vi "GINKGO - MTMP.vi"() -> ()   [LabVIEW 2015]
uses:
  Global Variable/GV_Z axis.vi
  Global Variable/GV_Lock State.vi
  <vilib>/FPGAPlugInAG/PXI-7854R/niLvFpga_Open_PXI-7854R.vi
  <vilib>/rvi/interface/common/dynamic/niFpgaDynamicAddResources.vi
  <vilib>/FPGAPlugInAG/PXIe-7962R/niLvFpga_Open_PXIe-7962R.vi
  <vilib>/FPGAPlugInAG/Dynamic/niLvFpga_Abort_Dynamic.vi
  <vilib>/FPGAPlugInAG/Dynamic/niLvFpga_Reset_Dynamic.vi
  <vilib>/rvi/interface/common/niFpgaWaitOnOcc.vi
  <vilib>/Utility/error.llb/Error Cluster From Error Code.vi
  <vilib>/FPGAPlugInAG/Dynamic/niLvFpga_Run_Dynamic.vi
  <vilib>/rvi/errors/niLvFpgaAdjustHostInterfaceError.vi
  <vilib>/FPGAPlugInAG/Dynamic/niLvFpga_Close_Dynamic.vi
  Controls/Save picture camera.vi
  <vilib>/rvi/interface/nirviOpenFPGA/nirviOpenFPGA.xnode
  FPGA Bitfiles/GINKGO-MTPM_7854R_FPGAControl5_ktnmj4hxrpw.lvbitx
  FPGA/FPGA Control.vi
  FPGA Bitfiles/GINKGO-MTPM_7962R_FPGA796xR3_DMzdrFahWxE.lvbitx
  FPGA/FPGA 796xR.vi
  <vilib>/rvi/interface/nirviMethod/nirviMethod.xnode
  <vilib>/rvi/interface/nirviReadWriteControl/nirviReadWriteControl.xnode
  <vilib>/rvi/interface/nirviCloseFPGA/nirviCloseFPGA.xnode
  <vilib>/rvi/interface/Simulation/niFpgaSimulationCallBeginRW.vi
  <vilib>/rvi/errors/niLvFpgaMergeErrorWithErrorCode.vi
  <vilib>/FPGAPlugInAG/Dynamic/niLvFpga_ReadFifo_Dynamic.vi
  <vilib>/FPGAPlugInAG/Dynamic/niLvFpga_StopFifo_Dynamic.vi
  <vilib>/vision/NI_Vision_Development_Module.lvlib
  <vilib>/FPGAPlugInAG/Dynamic/niLvFpga_WriteFifo_Dynamic.vi
  <vilib>/FPGAPlugInAG/Dynamic/niLvFpga_ConfigureFifo_Dynamic.vi
  NiFpgaLv.dll
  <vilib>/FPGAPlugInAG/Dynamic/niLvFpga_StartFifo_Dynamic.vi
  FPGA Bitfiles/GINKGO-MTPM_7853R_FPGAControl5_AQdVoJZ010M.lvbitx
  <vilib>/FPGAPlugInAG/PXI-7853R/niLvFpga_Open_PXI-7853R.vi
  FPGA Bitfiles/GINKGO-MTPM_7961R_FPGA796xR2_Co2ELON9TL0.lvbitx
  <vilib>/FPGAPlugInAG/PXIe-7961R/niLvFpga_Open_PXIe-7961R.vi
panel:
  out "波形图表":sgl(graph)=113.25391
  out "Power Stop":bool=TRUE
  in  "Rolling Queue Flag":bool=TRUE
  out "Total Data Out":u16=13612
  in  "Acq. Start":u16=38 caption="Phase" max=6000 step=1
  in  "Real Back Period":u16=5 min=1
  out "实际深度":u32=16777216
  in  "Map Max.":i32=10000 caption="Max."
  in  "Map Min.":i32=-1000 caption="Min."
  out "Scale Value":dbl=0.1 caption="X"
  out "Total Frames":u16=43366
  in  "Max. Min.":cluster{i32, i32}(slide)={2599, 200} scale=-1000.0..10000.0
  in  "16-bit Display Method":u32(ring)=14 caption="Display Method" items=["Full Dynamic"=12, "Given Range"=14]
  in  "Rolling Average":dbl=2.0 min=1.0 step=1.0
  in  "Rolling":bool=TRUE
  out "User Define Phase":u32=866
  out "Image":T1(plugin-control)
  in  "Controls":T2(tab)
  out "Offset value":i16=113
  in  "Read offset":bool
  in  "Start Device":bool
  in  "PMT Shutter Pow.":bool
  out "Overload Dis.":bool=TRUE
  in  "Pulse Number":enum16{"SP", "DP"}(ring)=enum."DP"
  in  "Mems Enable":bool
  out "中心偏移":i32
  in  "互相关点数":i32=5
  in  "Calculate Phase shift":bool
  in  "Wave":enum16{"Triangle", "Sine", "Ramp"}(ring)=enum."Sine"
  in  "Interval Dis.":sgl=0.00049965957 min=-10 max=50 format="%.4f"
  in  "stop z stage":bool
  in  "5V":bool
  in  "Voltage Level":dbl=15.0 format="%#.3p"
  in  "Voltage Level 2":dbl=-15.0 caption="Voltage Level" format="%#.3p"
  in  "Source:Output Enabled":bool
  out "Voltage Measurement 2":dbl=1.359809204859642e-05 caption="Voltage Measurement"
  out "Compliance/Limit Reached 2":bool caption="Compliance/Limit Reached"
  out "Voltage Measurement":i8
  out "Compliance/Limit Reached":bool
  in  "MEMS SLOW":dbl(slide)=240000.0 caption="Slow" min=0.0 max=1000000.0 step=100.0 scale=0.0..300000.0 scale format="%#_6p"
  in  "MEMS FAST":dbl(slide) caption="Fast" min=0.0 max=1000000.0 step=100.0 scale=0.0..300000.0 scale format="%#_6p"
  out "Stimulate Time Dis.":u32
  in  "Stimulate Value":dbl=5.0 min=-10.0 max=10.0 format="%#_3f"
  in  "Stimulate Time":u32=500
  out "Stimulate Interval Time":dbl=0.9846153846153847
  in  "Stimulate Interval":u32=10
  in  "Stimulate Enable":bool caption="V.S."
  out "Frame Befor Time":dbl=422889087.50769234
  out "Frame Number":u32=4294967295
  in  "Frames Befor Stimulate":u32
  out "Acq. Sample Rate":dbl=120000000.0 caption="Sanple Rate Divider" format="%#_6p"
  in  "Microscope":enum16{"Miniature", "Benchtop"}(ring)
  in  "Line":u32(ring)=512 caption="Y" items=["8"=8, "16"=16, "32"=32, "64"=64, "128"=128, "256"=256, "512"=512, "1024"=1024, "2048"=2048]
  in  "X Offset":dbl caption="X" format="%#_3f"
  in  "Y Offset":dbl caption="Y" min=-10.0 max=10.0 format="%#_3f"
  in  "X Frequency":dbl(slide)=2600.0 caption="Speed" min=50.0 max=10000.0 step=1.0 scale=0.0..5000.0
  in  "Laser Intensity":dbl(slide)=1.5168539325842696 max=10.0 scale=0.0..5.0
  in  "Phase Shift":u32(slide)=868 caption="Phase" max=15000 step=2 scale=0.0..15000.0
  in  "Point":bool
  in  "PMT1 Sensitivity":dbl(slide)=0.6500000000000001 min=0.0 max=0.95 step=0.05 scale=0.0..0.95 scale format="%#_3f"
  in  "PMT1 Enable":bool
  out "Pixel Dwell":dbl=0.2988 format="%#_3g"
  out "Actual Positon":sgl=11.119017
  out "Actual Laser Intensity":dbl(knob)=9.99969482421875 scale=-10.0..1.0
  in  "PMT2 Switch":bool
  in  "PMT2 Sensitivity":dbl(slide)=0.45 min=0.0 max=0.95 step=0.05 scale=0.0..0.95 scale format="%#_3f"
  in  "File Name":string
  in  "Scale":bool
  in  "XY Home":bool
  in  "XY UP":bool
  in  "XY DOWN":bool
  in  "XY LEFT":bool
  in  "XY RIGHT":bool
  in  "Stop":bool=TRUE
  in  "LIVE":bool
  in  "Save":bool
  in  "Z-Stack":bool
  in  "Pixel/Line":u16(ring)=512 caption="X" items=["8"=8, "16"=16, "32"=32, "64"=64, "128"=128, "256"=256, "512"=512, "1024"=1024, "2048"=2048]
  in  "Gain":enum16{"0dB", "6dB", "12dB"}(ring)
  in  "Coulple":enum16{"AC", "DC"}(ring)=enum."DC"
  in  "Path":path=path "C:/Users/TVS001/Desktop/DATA/20180327-FHIRM TPM-2/26-Aglight-3" caption="Images Folder"
  out "Save Frames Dis.":u16=100
  in  "Save Frames":u16=100
  in  "ZOOM":u16(ring)=1 items=["User Define", "1X", "1.5X", "2X", "2.5X", "3X", "3.5X", "4X", "4.5X", "5X", "6X"]
  in  "Scan Mode":enum16{"Normal", "Line Scan", "Random Access"}(ring)
  in  "Y Amplitude":dbl=0.6 caption="Y" min=-10.0 max=18.0 format="%0.2p"
  in  "X Amplitude":dbl=0.6 caption="X" min=-10.0 max=18.0 format="%.2p"
  in  "Add Phase":bool
  in  "Move":bool=TRUE
  out "Frame Rate":dbl=10.15625 format="%#_3g"
  out "Ready":u8(slide)=10 scale=0.0..10.0
  in  "Z":bool
  out "Position":sgl=-5.9652176 format="%#_6f"
  in  "Set Zero":bool caption="空白按钮"
  in  "Reset Zero":bool caption="空白按钮"
  in  "Home Z":bool
  in  "Abs. Go":bool
  in  "Abs Pos X":sgl min=-10 max=360 format="%.6f"
  in  "Z Up":bool
  in  "Z Down":bool
  in  "Jog":sgl=0.0005 caption="Z" min=0 max=50 step=0.0001 format="%.4f"
  in  "Frames/Slice":u16=5
  in  "Slices":u16=87
  out "End Dis.":sgl=0.043470383 format="%#_6f"
  out "Start Dis.":sgl format="%#_6f"
  in  "End":bool
  in  "Start":bool
  in  "Restart":bool
  in  "Interval Time":u32=150
  in  "Zoom Standard":dbl[][](array[numeric])=[[10.0, 10.0, 11251.0], [6.66, 6.66, 10603.0], [5.0, 5.0, 10394.0], [4.0, 4.0, 10394.0], [3.34, 3.34, 8602.0], [2.86, 2.86, 10394.0], [2.5, 2.5, 10394.0], [2.222, 2.222, 10394.0], [1.3, 1.3, 8294.0], [0.6, 0.6, 8296.0]]
  in  "Zoom Miniature":dbl[][](array[numeric])=[[14.0, 7.6, 868.0], [12.0, 7.0, 876.0], [9.0, 6.0, 876.0], [7.2, 5.6, 754.0], [5.0, 3.4, 738.0], [5.14, 4.0, 846.0], [4.0, 2.6, 858.0], [3.6, 2.0, 840.0], [3.2, 1.9, 872.0], [3.0, 1.9, 866.0]]
  out "Test Point 3":u32=227362
  out "Test Point":u32
  out "Point/Pixel":i32=36
  in  "Focus Flag":bool
  out "Queue Number":i32=2
  out "Initial Z":bool
  out "Initialization Done":bool=TRUE
  in  "Start Control":bool
  out "Memory":i32(slide) scale=0.0..5000.0
  in  "Resource Name":refnum<k15>="PXI1Slot6"
  in  "Channel Name":string="1" caption="Channel Name 1"
  in  "Current Limit":dbl=0.5 format="%.3p"
  in  "Voltage Level Range":dbl=20.0 format="%.5p"
  in  "Current Limit Range":dbl=1.0 format="%.3p"
  in  "Source Delay (Sec)":dbl=0.1 format="%.3p"
  in  "Channel Name 2":string="2"
  out "Current Measurement 2":dbl=-5.469513872563125e-06 caption="Current Measurement"
  out "Current Measurement":i16
  out "Actual DDS Ticks":u32=1
  out "Actual DDS Sample Freq":u32=279173
  in  "OUTPUT Value Ticks":u32=44
  in  "DDS Ticks":u32=1
  out "Actual OUTPUT Value Ticks":u32=44
  in  "Random 1D Array":fxp<+/-,32,16>[](array[numeric]) format="%.21g"
  in  "MG17Motor Z":refnum<k7>(container)
  out "Acq. Point Dis.":u16=32
  in  "Divide":enum16{"120M", "60M", "30M", "15M", "7.5M"}(ring)
  out "Nonlinear Acq.":bool=TRUE
  in  "Adapter Module User Data 1":u8
  in  "Adapter Module User Data 0":u8
  in  "Adapter Module User Command":u8=3
  in  "Apply":bool
  in  "HWSerialNum":i32=49871607
  in  "Set Large Scale":dbl=0.5 caption="X"
  in  "Set Small Scale":dbl=0.1 caption="X"
  in  "Set Zero Value":sgl format="%#_6f"
  in  "Fill Fraction":dbl=0.8 min=0.1 max=6.0 step=0.01
  in  "Back Period":u16=5 min=1
  in  "Initial Benchtop Speed":dbl=500.0 caption="Speed" min=50.0 max=10000.0 step=1.0
  in  "Initial Miniature Speed":dbl=2600.0 caption="Speed" min=50.0 max=10000.0 step=1.0
  out "Acq.Point Array":u16[](graph)=[38, 38, 38, 37, 37, 37, 37, 36, 36, 36, 36, 36, 35, 35, 35, 35, 35, 34, 34, 34, 34, 34, 34, 33, 33, 33, 33, 33, 33, 32, 32, 32, 32, 32, 32, 32, 32, 31, 31, 31, 31, 31, 31, 31, 31, 30, 30, 30, 30, 30, 30, 30, 30, 30, 30, 29, 29, 29, 29, 29, 29, 29, 29, 29, 29, 29, 28, 28, 28, 28, 28, 28, 28, 28, 28, 28, 28, 28, 28, 28, 27, 27, 27, 27, 27, 27, 27, 27, 27, 27, 27, 27, 27, 27, 27, 27, 26, 26, 26, 26, 26, 26, 26, 26, 26, 26, 26, 26, 26, 26, 26, 26, 26, 26, 26, 26, 26, 25, 25, 25, 25, 25, 25, 25, 25, 25, 25, 25, 25, 25, 25, 25, 25, 25, 25, 25, 25, 25, 25, 25, 25, 25, 25, 25, 24, 24, 24, 24, 24, 24, 24, 24, 24, 24, 24, 24, 24, 24, 24, 24, 24, 24, 24, 24, 24, 24, 24, 24, 24, 24, 24, 24, 24, 24, 24, 24, 24, 24, 24, 24, 24, 24, 24, 24, 24, 24, 24, 23, 23, 23, 23, 23, 23, 23, 23, 23, 23, 23, 23, 23, 23, 23, 23, 23, 23, 23, 23, 23, 23, 23, 23, 23, 23, 23, 23, 23, 23, 23, 23, 23, 23, 23, 23, 23, 23, 23, 23, 23, 23, 23, 23, 23, 23, 23, 23, 23, 23, 23, 23, 23, 23, 23, 23, 23, 23, 23, 23, 23, 23, 23, 23, 23, 23, 23, 23, 23, 23, 23, 23, 23, 23, 23, 23, 23, 23, 23, 23, 23, 23, 23, 23, 23, 23, 23, 23, 23, 23, 23, 23, 23, 23, 23, 23, 23, 23, 23, 23, 23, 23, 23, 23, 23, 23, 23, 23, 23, 23, 23, 23, 23, 23, 23, 23, 23, 23, 23, 23, 23, 23, 23, 23, 23, 23, 23, 23, 23, 23, 23, 23, 23, 23, 23, 23, 23, 23, 24, 24, 24, 24, 24, 24, 24, 24, 24, 24, 24, 24, 24, 24, 24, 24, 24, 24, 24, 24, 24, 24, 24, 24, 24, 24, 24, 24, 24, 24, 24, 24, 24, 24, 24, 24, 24, 24, 24, 24, 24, 24, 24, 25, 25, 25, 25, 25, 25, 25, 25, 25, 25, 25, 25, 25, 25, 25, 25, 25, 25, 25, 25, 25, 25, 25, 25, 25, 25, 25, 26, 26, 26, 26, 26, 26, 26, 26, 26, 26, 26, 26, 26, 26, 26, 26, 26, 26, 26, 26, 26, 27, 27, 27, 27, 27, 27, 27, 27, 27, 27, 27, 27, 27, 27, 27, 27, 28, 28, 28, 28, 28, 28, 28, 28, 28, 28, 28, 28, 28, 28, 29, 29, 29, 29, 29, 29, 29, 29, 29, 29, 29, 30, 30, 30, 30, 30, 30, 30, 30, 30, 30, 31, 31, 31, 31, 31, 31, 31, 31, 32, 32, 32, 32, 32, 32, 32, 32, 33, 33, 33, 33, 33, 33, 34, 34, 34, 34, 34, 34, 35, 35, 35, 35, 35, 36, 36, 36, 36, 36, 37, 37, 37, 37, 38, 38, 38]
  out "Init Data Out":u16[](array[numeric])=[38, 38, 38, 37, 37, 37, 37, 36, 36, 36, 36, 36, 35, 35, 35, 35, 35, 34, 34, 34, 34, 34, 34, 33, 33, 33, 33, 33, 33, 32, 32, 32, 32, 32, 32, 32, 32, 31, 31, 31, 31, 31, 31, 31, 31, 30, 30, 30, 30, 30, 30, 30, 30, 30, 30, 29, 29, 29, 29, 29, 29, 29, 29, 29, 29, 29, 28, 28, 28, 28, 28, 28, 28, 28, 28, 28, 28, 28, 28, 28, 27, 27, 27, 27, 27, 27, 27, 27, 27, 27, 27, 27, 27, 27, 27, 27, 26, 26, 26, 26, 26, 26, 26, 26, 26, 26, 26, 26, 26, 26, 26, 26, 26, 26, 26, 26, 26, 25, 25, 25, 25, 25, 25, 25, 25, 25, 25, 25, 25, 25, 25, 25, 25, 25, 25, 25, 25, 25, 25, 25, 25, 25, 25, 25, 24, 24, 24, 24, 24, 24, 24, 24, 24, 24, 24, 24, 24, 24, 24, 24, 24, 24, 24, 24, 24, 24, 24, 24, 24, 24, 24, 24, 24, 24, 24, 24, 24, 24, 24, 24, 24, 24, 24, 24, 24, 24, 24, 23, 23, 23, 23, 23, 23, 23, 23, 23, 23, 23, 23, 23, 23, 23, 23, 23, 23, 23, 23, 23, 23, 23, 23, 23, 23, 23, 23, 23, 23, 23, 23, 23, 23, 23, 23, 23, 23, 23, 23, 23, 23, 23, 23, 23, 23, 23, 23, 23, 23, 23, 23, 23, 23, 23, 23, 23, 23, 23, 23, 23, 23, 23, 23, 23, 23, 23, 23, 23, 23, 23, 23, 23, 23, 23, 23, 23, 23, 23, 23, 23, 23, 23, 23, 23, 23, 23, 23, 23, 23, 23, 23, 23, 23, 23, 23, 23, 23, 23, 23, 23, 23, 23, 23, 23, 23, 23, 23, 23, 23, 23, 23, 23, 23, 23, 23, 23, 23, 23, 23, 23, 23, 23, 23, 23, 23, 23, 23, 23, 23, 23, 23, 23, 23, 23, 23, 23, 23, 24, 24, 24, 24, 24, 24, 24, 24, 24, 24, 24, 24, 24, 24, 24, 24, 24, 24, 24, 24, 24, 24, 24, 24, 24, 24, 24, 24, 24, 24, 24, 24, 24, 24, 24, 24, 24, 24, 24, 24, 24, 24, 24, 25, 25, 25, 25, 25, 25, 25, 25, 25, 25, 25, 25, 25, 25, 25, 25, 25, 25, 25, 25, 25, 25, 25, 25, 25, 25, 25, 26, 26, 26, 26, 26, 26, 26, 26, 26, 26, 26, 26, 26, 26, 26, 26, 26, 26, 26, 26, 26, 27, 27, 27, 27, 27, 27, 27, 27, 27, 27, 27, 27, 27, 27, 27, 27, 28, 28, 28, 28, 28, 28, 28, 28, 28, 28, 28, 28, 28, 28, 29, 29, 29, 29, 29, 29, 29, 29, 29, 29, 29, 30, 30, 30, 30, 30, 30, 30, 30, 30, 30, 31, 31, 31, 31, 31, 31, 31, 31, 32, 32, 32, 32, 32, 32, 32, 32, 33, 33, 33, 33, 33, 33, 34, 34, 34, 34, 34, 34, 35, 35, 35, 35, 35, 36, 36, 36, 36, 36, 37, 37, 37, 37, 38, 38, 38]
  out "x amp. new":dbl
  out "y amp. new":dbl
  in  "Add Random Access":bool
  out "x offset new":i16=-7638
  out "y offset new":i16=-4030
  in  "All Random Array":fxp<+/-,32,16>[][](array[numeric])
  in  "Clear Array":bool
  out "Random Phase":u32=12 caption="Phase" max=6000 step=1
  # "File Name"
  # "File Path"
  # "Save Frames"
  # "Microscope"
  # "Scan Mode"
  # "PMT1"
  # "PMT2"
  # "Frame Size"
  # "Gain"
  # "Scan Speed"
  # "Hz"
  # "V"
  # "V"
  # "Rate"
  # "Frame Rate"
  # "μs"
  # "Hz"
  # "Pixel Dwell"
  # "XY"
  # "Z"
  # "Zoom"
  # "Point"
  # "Amplitude"
  # "V"
  # "V"
  # "Phase"
  # "Laser"
  # "Intensity Map"
  # "Recent Z"
  # "Frames Before"
  # "s"
  # "Stimulate Interval"
  # "s"
  # "ms"
  # "Stimulate Time"
  # "V"
  # "Stimulate Intensity"
  # "Mode Switch"
  # "MEMS Filter"
  # "Acquisition Mode"
  # "Image Settings"
  # "Magnification"
  # "Save Settings"
  # "Position Settings"
  # "Detection Settings"
  # "Z-scan Settings"
  # "Vision Stimulate Settings"
  # "X"
  # "Y"
  # "Phase"
  # "1X"
  # "1.5X"
  # "2X"
  # "2.5X"
  # "3X"
  # "3.5X"
  # "4X"
  # "4.5X"
  # "5X"
  # "6X"
  # "X"
  # "Y"
  # "Phase"
  # "1X"
  # "1.5X"
  # "2X"
  # "2.5X"
  # "3X"
  # "3.5X"
  # "4X"
  # "4.5X"
  # "5X"
  # "6X"
  # "40859011"
  # "83856379"
  # "AO0 -- X-Miniature  \nAO1 -- Y-Miniature\nAO2 -- Laser Intensity\nAO3 -- PMT1\nAO4 -- PMT2 \nAO5 -- \nAO6 -- X-Benchtop\nAO7 -- Y-Benchtop\n\nAI0  -- Actual Laser Intensity"
  # "DIO0 -- Acqusition  \nDIO1 -- VSYNC\nDIO2 -- HSYNC \nDIO3 -- Laser Shutter\nDIO4 -- MEMS FAST Filter\nDIO5 -- MEMS SLOW Filter\nDIO6 -- PMT Shutter\nDIO7 -- PMT Shutter Pow.\nDIO8 -- Shock Detection \nDIO9 -- Foot-plate LIVE Detection"
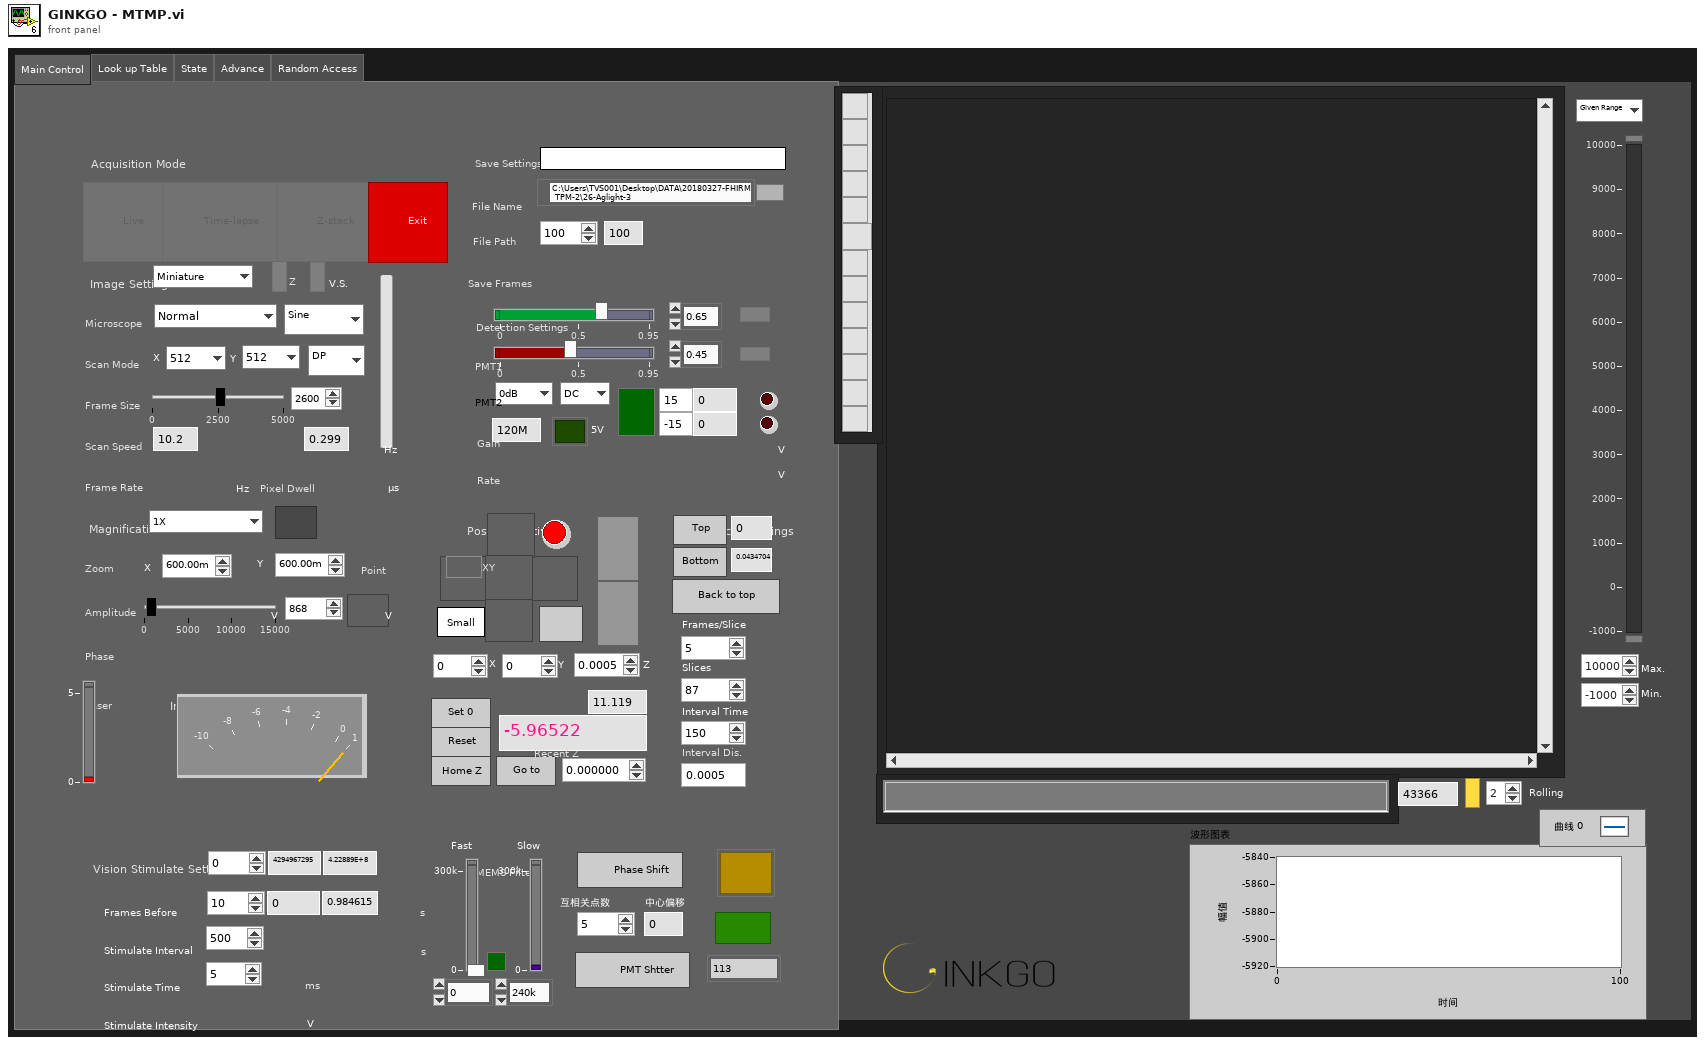
[diagram p1: front panel]
types:
  T1 = typedef "IMAQ Image.ctl" = refnum<image>
  T2 = enum32{"Main Control", "Look up Table", "State", "Advance", "Random Access"}
  T3 = typedef "Image Type" = u32
  T4 = enum8{"Enabled", "Disabled", "Disabled and Grayed Out"}
  T5 = cluster{"Global Rectangle":i32[], "Contours":cluster{"Contour Type":u32, "ROI Type":u32, "Points":i32[]}[]}
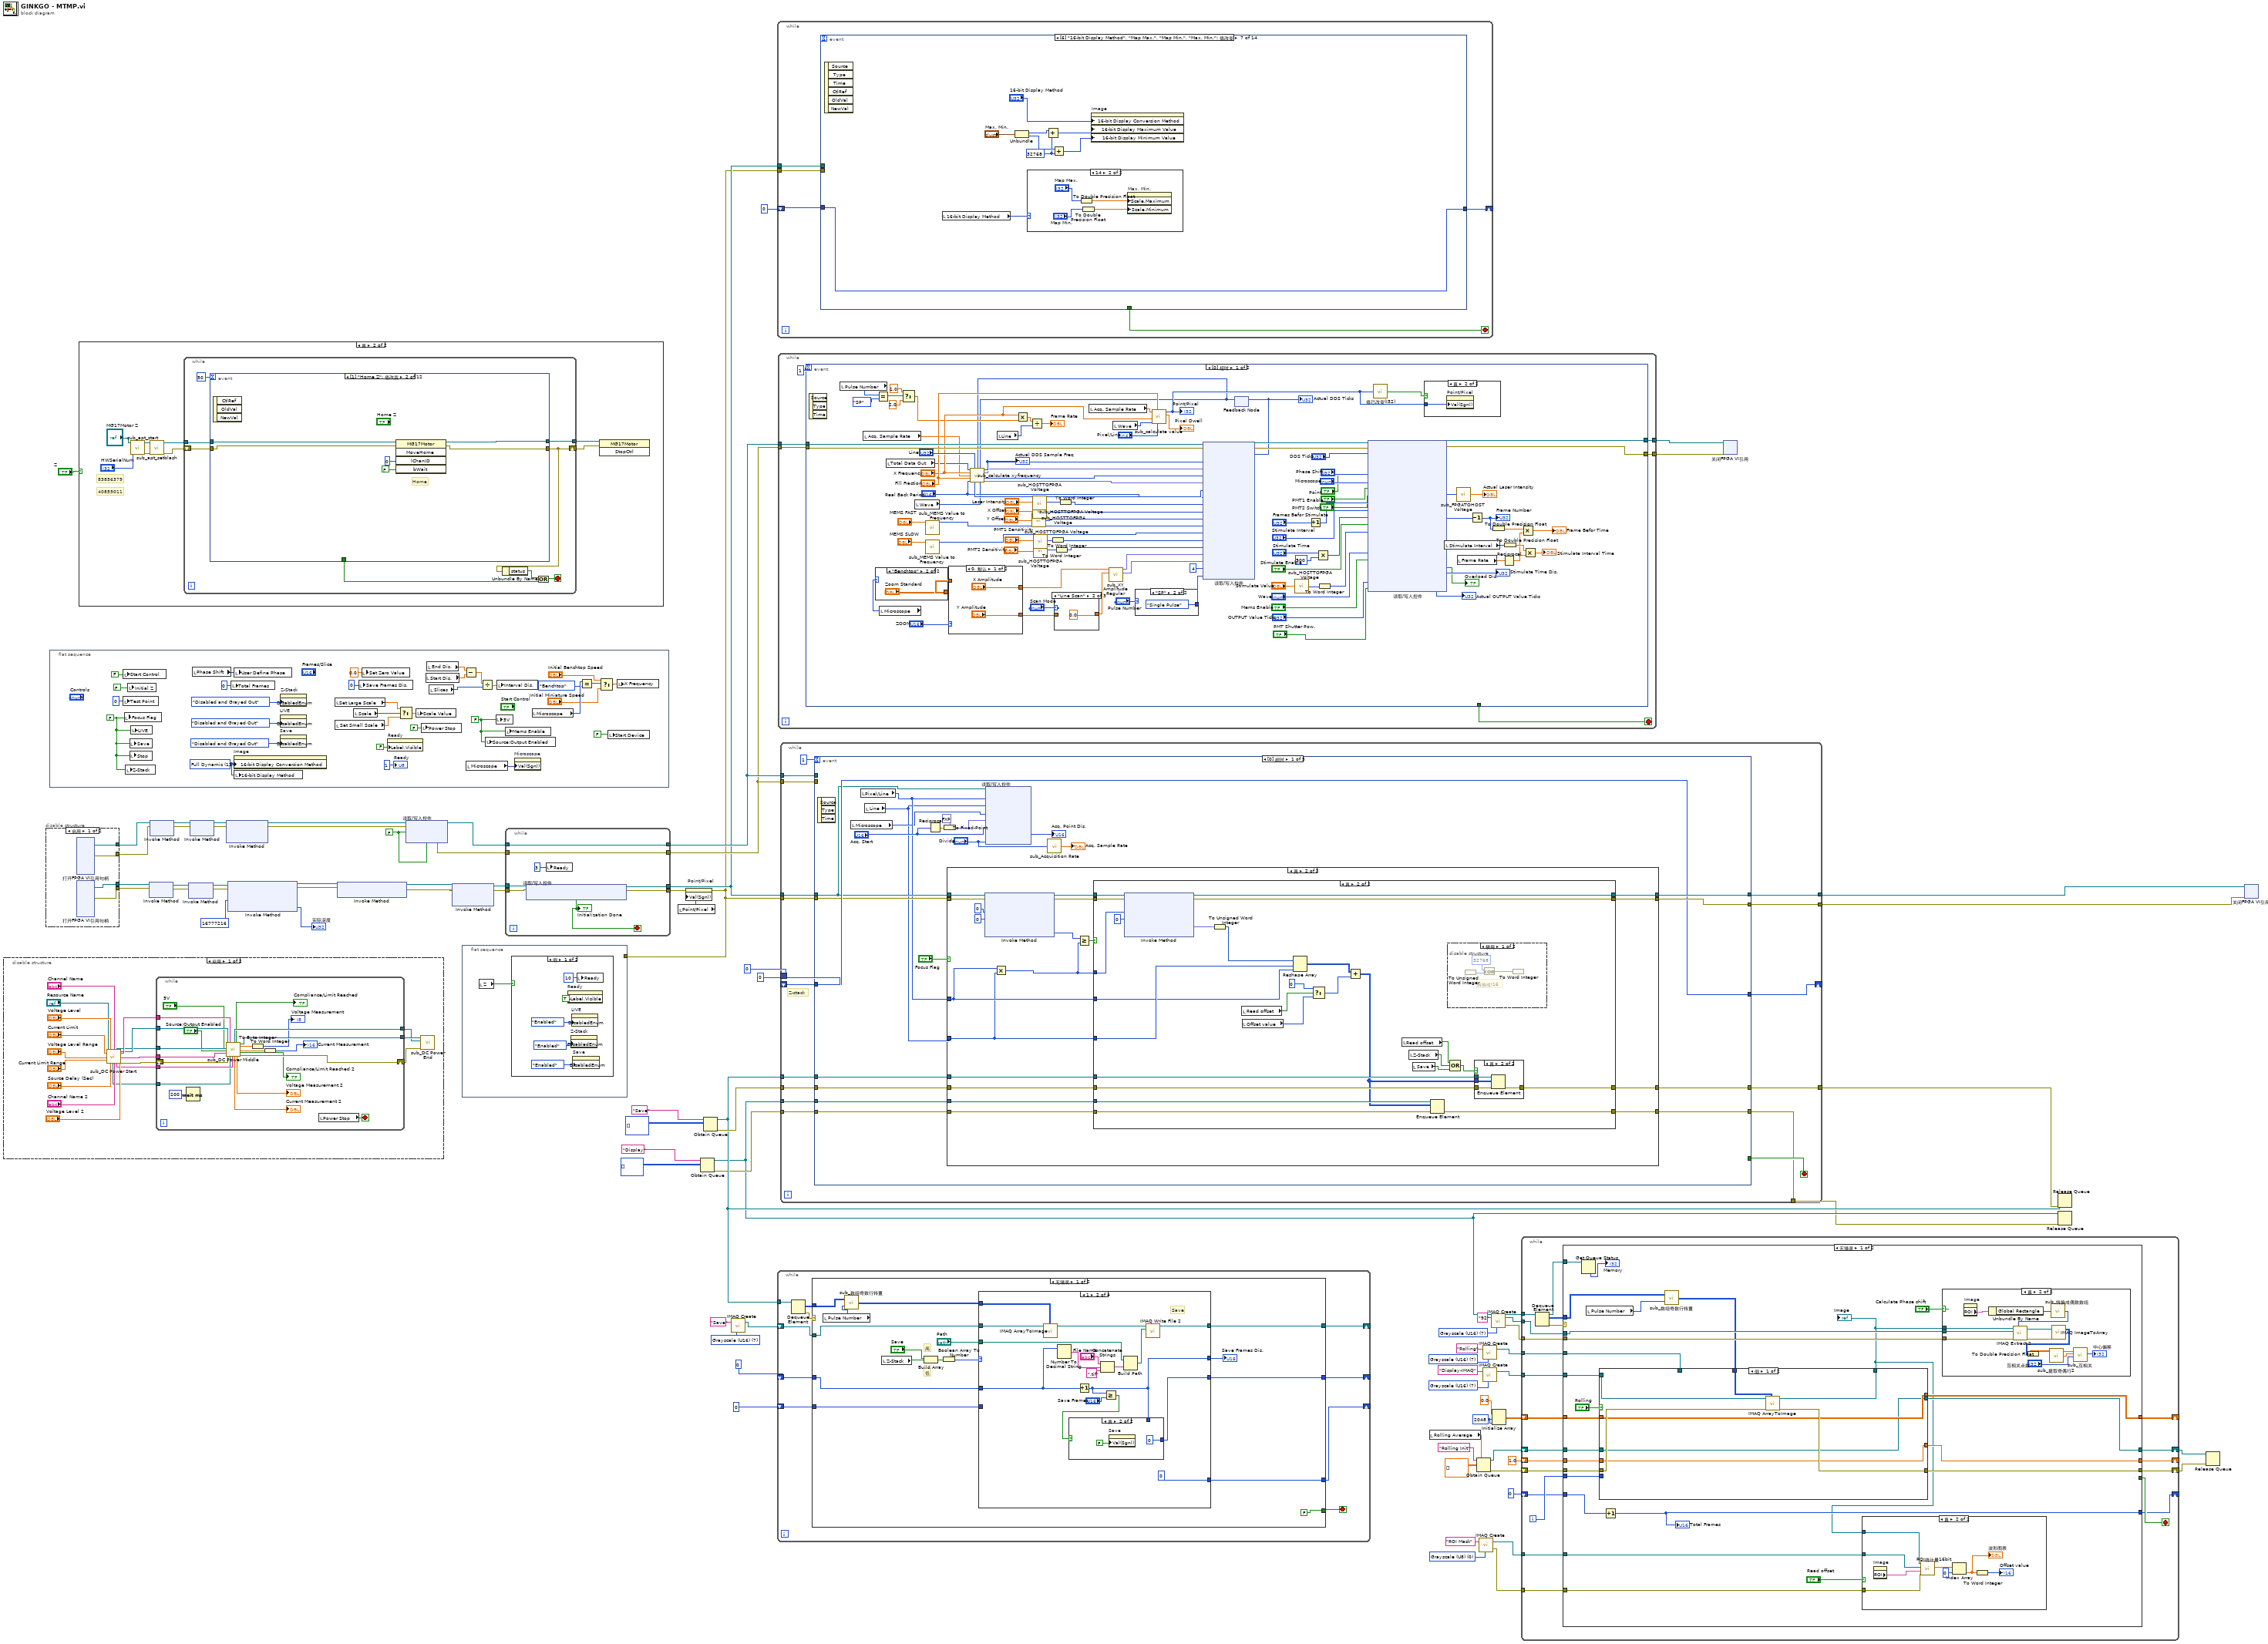
[diagram p0: block diagram]
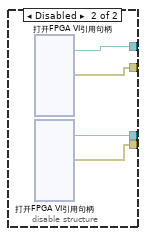
[diagram p2: hidden frame]
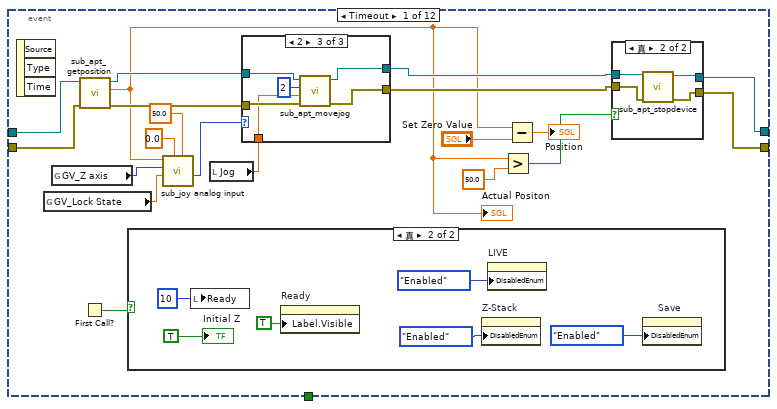
[diagram p4: hidden frame]
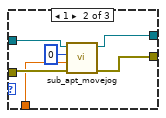
[diagram p6: hidden frame]
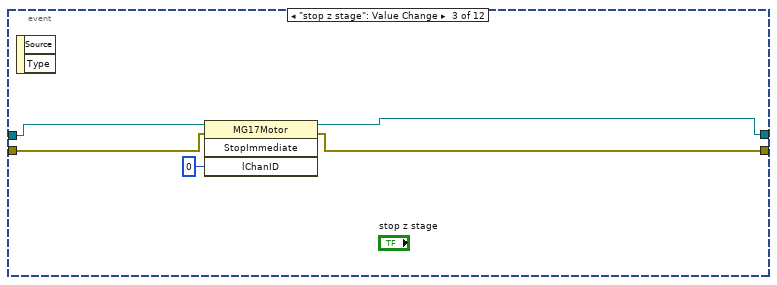
[diagram p9: hidden frame]
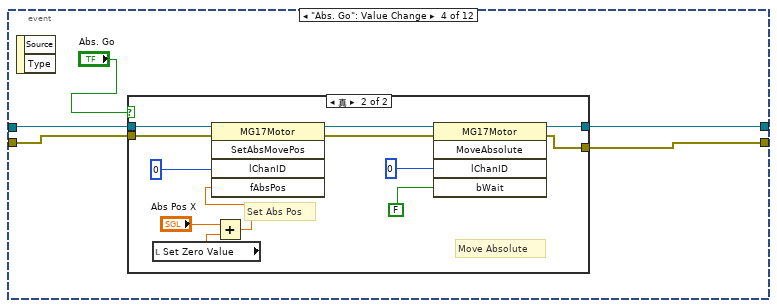
[diagram p10: hidden frame]
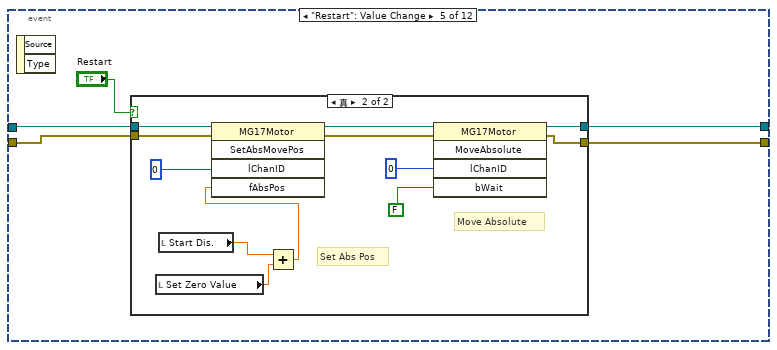
[diagram p12: hidden frame]
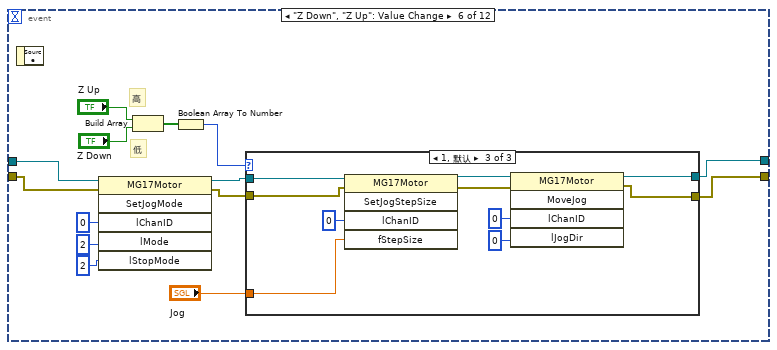
[diagram p14: hidden frame]
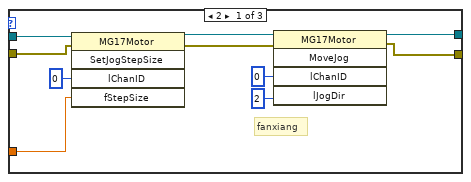
[diagram p15: hidden frame]
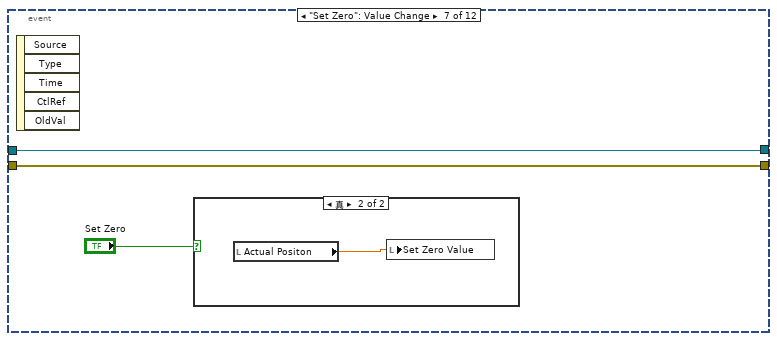
[diagram p17: hidden frame]
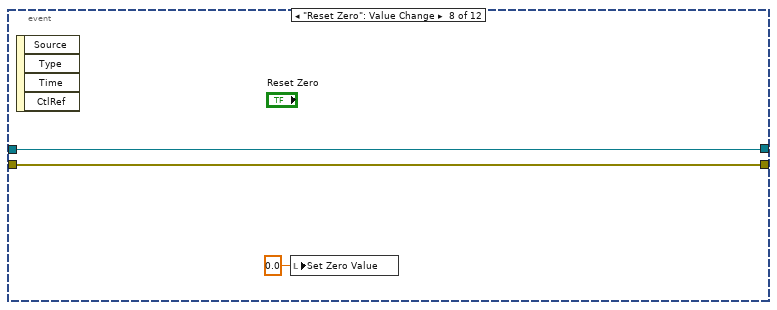
[diagram p19: hidden frame]
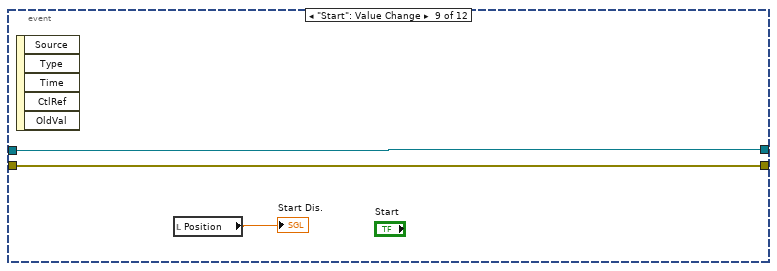
[diagram p20: hidden frame]
diagram:
  w3 = T3 0 items=["Grayscale (U8)", "Grayscale (I16)", "Grayscale (SGL)", "Complex (CSG)", "RGB (U32)", "HSL (U32)", "RGB (U64)", "Grayscale (U16)"] ("Image Type")
  w9 = T3 7 items=["Grayscale (U8)", "Grayscale (I16)", "Grayscale (SGL)", "Complex (CSG)", "RGB (U32)", "HSL (U32)", "RGB (U64)", "Grayscale (U16)"] ("Image Type")
  w15 = T3 7 items=["Grayscale (U8)", "Grayscale (I16)", "Grayscale (SGL)", "Complex (CSG)", "RGB (U32)", "HSL (U32)", "RGB (U64)", "Grayscale (U16)"] ("Image Type")
  w28 = T3 7 items=["Grayscale (U8)", "Grayscale (I16)", "Grayscale (SGL)", "Complex (CSG)", "RGB (U32)", "HSL (U32)", "RGB (U64)", "Grayscale (U16)"] ("Image Type")
  w38 = 2048 ("维数大小")
  w35 = T3 7 items=["Grayscale (U8)", "Grayscale (I16)", "Grayscale (SGL)", "Complex (CSG)", "RGB (U32)", "HSL (U32)", "RGB (U64)", "Grayscale (U16)"] ("Image Type")
  w49 = FALSE ("Enable")
  n1 = disable-structure shown="启用" {
    frame Enabled {
      n2 = call "sub_DC Power Start.vi"("IVI引用句柄输入"="Resource Name", "Current Limit"="Current Limit", "Voltage Level Range"="Voltage Level Range", "Current Limit Range"="Current Limit Range", "Voltage Level"="Voltage Level", "Source Delay (Sec)"="Source Delay (Sec)", "Channel Name"="Channel Name", "Channel Name 2"="Channel Name 2", "Voltage Level 2"="Voltage Level 2") -> ("instrument handle out 2"=w81:refnum<k15>, "instrument handle out"=w88:refnum<k15>, "Channel Name 6"=w82:string, "IVI引用句柄输出"=w96:refnum<k15>, "Channel Name 4"=w97:string, "Channel Name 3"=w90:string, "错误输出"=w87:errorcluster)  [unwired: 4 in]
      n3 = while {
        tunnel: w97 -> [w121]
        tunnel: w90 -> [w120]
        tunnel: [w119] -> w89
        shift-right: [w118] -> w86
        shift-left: w87 -> [w115]
        tunnel: w88 -> [w114]
        tunnel: w96 -> [w116]
        tunnel: [w117] -> w98
        tunnel: w82 -> [w104]
        tunnel: w81 -> [w103]
        stop <- w105 stop-if-true
        n4 = Wait (ms)(milliseconds to wait=u32 200 ("等待时间（毫秒）")) -> ()  [unwired: 1 out]
        n5 = call "sub_DC Power Middle.vi"("IVI引用句柄输入"=w116, "instrument handle out"=w114, "5V"="5V", "Source:Output Enabled"="Source:Output Enabled", "Channel Name 3"=w120, "错误输入（无错误）"=w115, "Channel Name 4"=w121, "instrument handle out 2"=w103, "Channel Name 5"=w104) -> ("instrument handle out 3"=w119:refnum<k15>, "Current Measurement 2"=→"Current Measurement 2":dbl, "Compliance/Limit Reached"=→"Compliance/Limit Reached":bool, "Voltage Measurement 2"=→"Voltage Measurement 2":dbl, "IVI引用句柄输出"=w117:refnum<k15>, "Voltage Measurement"=w111:dbl, "Current Measurement"=w110:dbl, "Compliance/Limit Reached 2"=→"Compliance/Limit Reached 2":bool, "错误输出"=w118:errorcluster)  [unwired: 2 in]
        n6 = To Byte Integer(number=w111) -> (8bit integer=→"Voltage Measurement":i8)
        n7 = To Word Integer(number=w110) -> (16bit integer=→"Current Measurement":i16)
        n8 = local read "Power Stop"() -> (w105:bool)
      }
      n9 = call "sub_DC Power End.vi"("错误输入（无错误）"=w86, "instrument handle out"=w89, "IVI引用句柄输入"=w98) -> ()  [unwired: 9 in]
    }
    frame Disabled {
    }
  }
  n10 = disable-structure shown="启用" {
    disable-tunnel: [w125 w129] -> w80
    disable-tunnel: [w124 w128] -> w79
    disable-tunnel: [w123 w126] -> w78
    disable-tunnel: [w122 w127] -> w77
    frame Enabled {
      n11 = xnode "打开FPGA VI引用句柄"() -> ("FPGA VI引用输出"=w125:refnum<k20>, "错误输出"=w124:errorcluster)  [unwired: 2 in]
      n12 = xnode "打开FPGA VI引用句柄"() -> ("FPGA VI引用输出"=w122:refnum<k20>, "错误输出"=w123:errorcluster)  [unwired: 2 in]
    }
    frame Disabled {
      n13 = xnode "打开FPGA VI引用句柄"() -> ("FPGA VI引用输出"=w129:refnum<k20>, "错误输出"=w128:errorcluster)  [unwired: 2 in]
      n14 = xnode "打开FPGA VI引用句柄"() -> ("FPGA VI引用输出"=w127:refnum<k20>, "错误输出"=w126:errorcluster)  [unwired: 2 in]
    }
  }
  n15 = flat-sequence {
    frame #0 {
      w144 = FALSE ("Focus")
      w152 = u32 12 items=["Default"=10, "Most Significant Bits"=11, "Full Dynamic"=12, "Downshift"=13, "Given Range"=14, "90% Dynamic"=15, "Given Percent Range"=16] ("16-bit Display Mapping:Conversion Method")
      w159 = FALSE ("Focus")
      n16 = local write "Start Control"(FALSE ("Initial")) -> ()
      n17 = local write "Test Point"(u32 0 ("Test Point")) -> ()
      n18 = local write "Focus Flag"(w159) -> ()
      n19 = local write "Z-Stack"(w159) -> ()
      n20 = local write "Initial Z"(FALSE ("Initial")) -> ()
      n21 = local write "Save"(w159) -> ()
      n22 = local write "Stop"(w159) -> ()
      n23 = local write "LIVE"(w159) -> ()
      n24 = local read "Phase Shift"() -> (w145:u32)
      n25 = local write "Total Frames"(u16 0 ("Total Frames")) -> ()
      n26 = property on="Image" class="ImageControl"("16-bit Display Conversion Method"=w152) -> ()  [unwired: 2 in, 2 out]
      n27 = local write "User Define Phase"(w145) -> ()
      n28 = local write "16-bit Display Method"(w152) -> ()
      n29 = property on="LIVE" class="Bool (严格)"("DisabledEnum"=T4."Disabled and Grayed Out" ("禁用")) -> ()  [unwired: 2 in, 2 out]
      n30 = property on="Save" class="Bool (严格)"("DisabledEnum"=T4."Disabled and Grayed Out" ("禁用")) -> ()  [unwired: 2 in, 2 out]
      n31 = property on="Z-Stack" class="Bool (严格)"("DisabledEnum"=T4."Disabled and Grayed Out" ("禁用")) -> ()  [unwired: 2 in, 2 out]
      n32 = local read "Set Large Scale"() -> (w151:dbl)
      n33 = local read "Set Small Scale"() -> (w150:dbl)
      n34 = local read "Scale"() -> (w149:bool)
      n35 = local write "Save Frames Dis."(u16 0 ("Save Frames Dis.")) -> ()
      n36 = local write "Set Zero Value"(sgl 0.0 ("Set Zero Value")) -> ()
      n37 = property on="Ready" class="Slide (严格)"("Label.Visible"=FALSE ("标签.可见")) -> ()  [unwired: 2 in, 2 out]
      n38 = Select(t=w151, s=w149, f=w150) -> (s? t:f=w148:dbl)
      n39 = local write "Scale Value"(w148) -> ()
      n40 = local write "Power Stop"(FALSE ("Power Stop")) -> ()
      n41 = local read "Start Dis."() -> (w141:sgl)
      n42 = local read "End Dis."() -> (w140:sgl)
      n43 = local read "Slices"() -> (w139:u16)
      n44 = Subtract(x=w140, y=w141) -> (x-y=w142:sgl)
      n45 = local read "Microscope"() -> (w138:enum16{"Miniature", "Benchtop"})
      n46 = Divide(x=w142, y=w139) -> (x/y=w143:sgl)
      n47 = local write "Source:Output Enabled"(w144) -> ()
      n48 = local write "5V"(w144) -> ()
      n49 = local write "Interval Dis."(w143) -> ()
      n50 = local write "Mems Enable"(w144) -> ()
      n51 = property on="Microscope" class="Enum (严格)"("Val(Sgnl)"=w138) -> ()  [unwired: 2 in, 2 out]
      n52 = local read "Microscope"() -> (w136:enum16{"Miniature", "Benchtop"})
      n53 = Equal?(x=w136, y=enum16{"Miniature", "Benchtop"}."Benchtop") -> (x = y?=w135:bool)
      n54 = Select(t="Initial Benchtop Speed", s=w135, f="Initial Miniature Speed") -> (s? t:f=w133:dbl)
      n55 = local write "Start Device"(FALSE ("Start Device")) -> ()
      n56 = local write "X Frequency"(w133) -> ()
      "Ready" <- u8 1 ("Process")
    }
  }
  n57 = case shown="真" "Z" {
    frame False {
    }
    frame True {
      # "40859011"
      # "83856379"
      n58 = call "sub_apt_start.vi"("HWSerialNum"="HWSerialNum", "引用"="MG17Motor Z") -> ("错误输出"=w167:errorcluster, "引用输出"=w168:refnum<k7>)  [unwired: 8 in]
      n59 = call "sub_apt_setblash.vi"("错误输入（无错误）"=w167, "引用"=w168) -> ("错误输出"=w165:errorcluster, "引用输出"=w166:refnum<k7>)  [unwired: 8 in]
      n60 = while {
        shift-right: [w174] -> w169
        shift-left: w165 -> [w177]
        tunnel: w166 -> [w178]
        tunnel: [w176] -> w170
        stop <- w172 stop-if-true
        n61 = event shown="[1] \"Home Z\": 值改变" {
          selector: _ -> [_ _ _ _ _ _ _ _ _ _ _ _]
          dyn-events: _ -> [_ _ _ _ _ _ _ _ _ _ _ _]
          timeout: 50 -> [_ _ _ _ _ _ _ _ _ _ _ _]
          tunnel: w178 -> [w191 w226 w234 w240 w259 w279 w312 w316 w319 w322 w325 w358]
          tunnel: w177 -> [w190 w225 w233 w239 w258 w278 w311 w315 w318 w321 w324 w357]
          tunnel: [w196 w228 w232 w238 w257 w287 w312 w316 w319 w322 w334 w358] -> w176
          tunnel: [w195 w227 w231 w237 w256 w286 w311 w315 w318 w321 w333 w357] -> w174
          tunnel: [_ _ _ _ _ _ _ _ _ _ _ TRUE ("Stop")] -> w171
          event Timeout {
            n62 = event-data() -> ()  [unwired: 1 in, 3 out]
            n63 = global read "GV_Lock State.vi" "GV_Lock State"() -> (w180:dbl)
            n64 = global read "GV_Z axis.vi" "GV_Z axis"() -> (w181:i32)
            n65 = call "sub_apt_getposition.vi"("错误输入（无错误）"=w190, "引用"=w191) -> ("错误输出"=w187:errorcluster, "GetPosition_Position"=w182:sgl, "引用输出"=w188:refnum<k7>)  [unwired: 7 in]
            "Actual Positon" <- w182
            n66 = First Call?() -> (First Call?: T/F=w194:bool)
            n67 = case shown="真" w194 {
              frame False {
              }
              frame True {
                n68 = local write "Ready"(u8 10 ("Process")) -> ()
                n69 = property on="Ready" class="Slide (严格)"("Label.Visible"=TRUE ("标签.可见")) -> ()  [unwired: 2 in, 2 out]
                n70 = property on="Z-Stack" class="Bool (严格)"("DisabledEnum"=T4."Enabled" ("禁用")) -> ()  [unwired: 2 in, 2 out]
                n71 = property on="LIVE" class="Bool (严格)"("DisabledEnum"=T4."Enabled" ("禁用")) -> ()  [unwired: 2 in, 2 out]
                n72 = property on="Save" class="Bool (严格)"("DisabledEnum"=T4."Enabled" ("禁用")) -> ()  [unwired: 2 in, 2 out]
                "Initial Z" <- TRUE ("Initial")
              }
            }
            n73 = call "sub_joy analog input.vi"("上限"=50.0 ("Displacement"), "下限"=0.0 ("Displacement"), "lock输入奇偶"=w180, "x"=w181, "Displacement"=w182) -> ("x state"=w183:i32)  [unwired: 5 in, 1 out]
            n74 = local read "Jog"() -> (w179:sgl)
            n75 = case shown="2" w183 {
              tunnel: [w200 w203 w209] -> w189
              tunnel: w188 -> [w200 w206 w212]
              tunnel: w187 -> [w199 w205 w211]
              tunnel: [w199 w204 w210] -> w186
              tunnel: w179 -> [_ w202 w208]
              frame 0, Default {
              }
              frame 1 {
                n76 = call "sub_apt_movejog.vi"("错误输入（无错误）"=w205, "Rel. Pos Y"=w202, "lJogDir"=0, "引用"=w206) -> ("error out"=w204:errorcluster, "MG17Motor Y"=w203:refnum<k7>)  [unwired: 6 in]
              }
              frame 2 {
                n77 = call "sub_apt_movejog.vi"("错误输入（无错误）"=w211, "Rel. Pos Y"=w208, "lJogDir"=2, "引用"=w212) -> ("error out"=w210:errorcluster, "MG17Motor Y"=w209:refnum<k7>)  [unwired: 6 in]
              }
            }
            n78 = Greater?(x=w182, y=sgl 50.0) -> (0:w197:bool)
            n79 = Subtract(x=w182, y="Set Zero Value") -> (x-y=→"Position":sgl)
            n80 = case shown="真" w197 {
              tunnel: w189 -> [w220 w224]
              tunnel: w186 -> [w219 w223]
              tunnel: [w220 w222] -> w196
              tunnel: [w219 w221] -> w195
              frame False {
              }
              frame True {
                n81 = call "sub_apt_stopdevice.vi"("错误输入（无错误）"=w223, "引用"=w224) -> ("错误输出"=w221:errorcluster, "引用输出"=w222:refnum<k7>)  [unwired: 8 in]
              }
            }
          }
          event "Home Z": Value Change {
            # "Home"
            n82 = event-data() -> ()  [unwired: 1 in, 3 out]
            n83 = invoke class="MG17Motor" method="MoveHome"(reference=w226, error in=w225, "lChanID"=0, "bWait"=FALSE) -> (reference out=w228:refnum<k7>, error out=w227:errorcluster)  [unwired: 1 in, 3 out]
          }
          event "stop z stage": Value Change {
            n84 = event-data() -> ()  [unwired: 1 in, 2 out]
            n85 = invoke class="MG17Motor" method="StopImmediate"(reference=w234, error in=w233, "lChanID"=0) -> (reference out=w232:refnum<k7>, error out=w231:errorcluster)  [unwired: 1 in, 2 out]
          }
          event "Abs. Go": Value Change {
            n86 = event-data() -> ()  [unwired: 1 in, 2 out]
            n87 = case shown="真" "Abs. Go" {
              tunnel: w240 -> [w242 w251]
              tunnel: w239 -> [w241 w250]
              tunnel: [w242 w247] -> w238
              tunnel: [w241 w246] -> w237
              frame False {
              }
              frame True {
                # "Set Abs Pos"
                # "Move Absolute"
                n88 = local read "Set Zero Value"() -> (w244:sgl)
                n89 = Add(x="Abs Pos X", y=w244) -> (x+y=w243:sgl)
                n90 = invoke class="MG17Motor" method="SetAbsMovePos"(reference=w251, error in=w250, "lChanID"=0, "fAbsPos"=w243) -> (reference out=w249:refnum<k7>, error out=w248:errorcluster)  [unwired: 1 in, 3 out]
                n91 = invoke class="MG17Motor" method="MoveAbsolute"(reference=w249, error in=w248, "lChanID"=0, "bWait"=FALSE) -> (reference out=w247:refnum<k7>, error out=w246:errorcluster)  [unwired: 1 in, 3 out]
              }
            }
          }
          event "Restart": Value Change {
            n92 = event-data() -> ()  [unwired: 1 in, 2 out]
            n93 = case shown="真" "Restart" {
              tunnel: w259 -> [w261 w270]
              tunnel: w258 -> [w260 w269]
              tunnel: [w261 w266] -> w257
              tunnel: [w260 w265] -> w256
              frame False {
              }
              frame True {
                # "Set Abs Pos"
                # "Move Absolute"
                n94 = local read "Set Zero Value"() -> (w264:sgl)
                n95 = local read "Start Dis."() -> (w263:sgl)
                n96 = Add(x=w263, y=w264) -> (x+y=w262:sgl)
                n97 = invoke class="MG17Motor" method="SetAbsMovePos"(reference=w270, error in=w269, "lChanID"=0, "fAbsPos"=w262) -> (reference out=w268:refnum<k7>, error out=w267:errorcluster)  [unwired: 1 in, 3 out]
                n98 = invoke class="MG17Motor" method="MoveAbsolute"(reference=w268, error in=w267, "lChanID"=0, "bWait"=FALSE) -> (reference out=w266:refnum<k7>, error out=w265:errorcluster)  [unwired: 1 in, 3 out]
              }
            }
          }
          event "Z Down", "Z Up": Value Change {
            # "低"
            # "高"
            n99 = event-data() -> ()  [unwired: 1 in, 1 out]
            n100 = invoke class="MG17Motor" method="SetJogMode"(reference=w279, error in=w278, "lChanID"=0, "lMode"=2, "lStopMode"=2) -> (reference out=w281:refnum<k7>, error out=w280:errorcluster)  [unwired: 1 in, 4 out]
            n101 = Build Array("Z Up", "Z Down") -> (w283:bool[])
            n102 = Boolean Array To Number(Boolean array=w283) -> (number=w282:u32)
            n103 = case shown="1, 默认" w282 {
              tunnel: w281 -> [w297 w299 w309]
              tunnel: [w295 w299 w307] -> w287
              tunnel: w280 -> [w292 w298 w304]
              tunnel: [w290 w298 w302] -> w286
              tunnel: "Jog" -> [w288 _ w300]
              frame 2 {
                # "fanxiang"
                n104 = invoke class="MG17Motor" method="SetJogStepSize"(reference=w297, error in=w292, "lChanID"=0, "fStepSize"=w288) -> (reference out=w296:refnum<k7>, error out=w291:errorcluster)  [unwired: 1 in, 3 out]
                n105 = invoke class="MG17Motor" method="MoveJog"(reference=w296, error in=w291, "lChanID"=0, "lJogDir"=2) -> (reference out=w295:refnum<k7>, error out=w290:errorcluster)  [unwired: 1 in, 3 out]
              }
              frame 0 {
              }
              frame 1, Default {
                n106 = invoke class="MG17Motor" method="SetJogStepSize"(reference=w309, error in=w304, "lChanID"=0, "fStepSize"=w300) -> (reference out=w308:refnum<k7>, error out=w303:errorcluster)  [unwired: 1 in, 3 out]
                n107 = invoke class="MG17Motor" method="MoveJog"(reference=w308, error in=w303, "lChanID"=0, "lJogDir"=0) -> (reference out=w307:refnum<k7>, error out=w302:errorcluster)  [unwired: 1 in, 3 out]
              }
            }
          }
          event "Set Zero": Value Change {
            n108 = event-data() -> ()  [unwired: 1 in, 5 out]
            n109 = case shown="真" "Set Zero" {
              frame False {
              }
              frame True {
                n110 = local read "Actual Positon"() -> (w313:sgl)
                n111 = local write "Set Zero Value"(w313) -> ()
              }
            }
          }
          event "Reset Zero": Value Change {
            n112 = event-data() -> ()  [unwired: 1 in, 4 out]
            n113 = local write "Set Zero Value"(sgl 0.0 ("Set Zero Value")) -> ()
          }
          event "Start": Value Change {
            n114 = event-data() -> ()  [unwired: 1 in, 5 out]
            n115 = local read "Position"() -> (→"Start Dis.":sgl)
          }
          event "End": Value Change {
            n116 = event-data() -> ()  [unwired: 1 in, 3 out]
            n117 = local read "Position"() -> (→"End Dis.":sgl)
          }
          event "Move": Value Change {
            n118 = event-data() -> ()  [unwired: 1 in, 1 out]
            n119 = invoke class="MG17Motor" method="SetJogMode"(reference=w325, error in=w324, "lChanID"=0, "lMode"=2, "lStopMode"=2) -> (reference out=w326:refnum<k7>, error out=w323:errorcluster)  [unwired: 1 in, 4 out]
            n120 = Absolute Value(x="Interval Dis.") -> (abs(x)=w330:sgl)
            n121 = Greater Than 0?(x="Interval Dis.") -> (x > 0?=w331:bool)
            n122 = case shown="假" w331 {
              tunnel: w326 -> [w346 w356]
              tunnel: [w344 w354] -> w334
              tunnel: w323 -> [w341 w351]
              tunnel: [w339 w349] -> w335
              tunnel: w330 -> [w337 w347]
              frame False {
                # "fanxiang"
                n123 = invoke class="MG17Motor" method="SetJogStepSize"(reference=w346, error in=w341, "lChanID"=0, "fStepSize"=w337) -> (reference out=w345:refnum<k7>, error out=w340:errorcluster)  [unwired: 1 in, 3 out]
                n124 = invoke class="MG17Motor" method="MoveJog"(reference=w345, error in=w340, "lChanID"=0, "lJogDir"=2) -> (reference out=w344:refnum<k7>, error out=w339:errorcluster)  [unwired: 1 in, 3 out]
              }
              frame True {
                n125 = invoke class="MG17Motor" method="SetJogStepSize"(reference=w356, error in=w351, "lChanID"=0, "fStepSize"=w347) -> (reference out=w355:refnum<k7>, error out=w350:errorcluster)  [unwired: 1 in, 3 out]
                n126 = invoke class="MG17Motor" method="MoveJog"(reference=w355, error in=w350, "lChanID"=0, "lJogDir"=0) -> (reference out=w354:refnum<k7>, error out=w349:errorcluster)  [unwired: 1 in, 3 out]
              }
            }
            n127 = property on="Z-Stack" class="Bool (严格)"(error in=w335, "Val(Sgnl)"=TRUE ("值(信号)")) -> (error out=w333:errorcluster)  [unwired: 1 in, 1 out]
          }
          event "Stop": Value Change {
            n128 = event-data() -> ()  [unwired: 1 in, 4 out]
          }
        }
        n129 = Unbundle By Name(w174) -> ("status"=w173:bool)
        n130 = Or(x=w173, y=w171) -> (x .or. y?=w172:bool)
      }
      n131 = invoke class="MG17Motor" method="StopCtrl"(reference=w170, error in=w169) -> ()  [unwired: 1 in, 3 out]
    }
  }
  n132 = xnode "Invoke Method"("FPGA VI引用输入"=w77, "错误输入"=w78) -> ("FPGA VI引用输出"=w66:refnum<k20>, "错误输出"=w67:errorcluster)
  n133 = xnode "Invoke Method"("FPGA VI引用输入"=w80, "错误输入"=w79) -> ("FPGA VI引用输出"=w63:refnum<k20>, "错误输出"=w62:errorcluster)
  n134 = xnode "Invoke Method"("FPGA VI引用输入"=w66, "错误输入"=w67) -> ("FPGA VI引用输出"=w68:refnum<k20>, "错误输出"=w69:errorcluster)
  n135 = xnode "Invoke Method"("FPGA VI引用输入"=w63, "错误输入"=w62) -> ("FPGA VI引用输出"=w61:refnum<k20>, "错误输出"=w60:errorcluster)
  n136 = xnode "Invoke Method"("FPGA VI引用输入"=w61, "错误输入"=w60) -> ("FPGA VI引用输出"=w59:refnum<k20>, "错误输出"=w58:errorcluster)  [unwired: 1 in]
  n137 = xnode "Invoke Method"("FPGA VI引用输入"=w68, "错误输入"=w69, "请求的深度"=u32 16777216) -> ("FPGA VI引用输出"=w65:refnum<k20>, "错误输出"=w64:errorcluster, "实际深度"=→"实际深度":u32)
  n138 = xnode "Invoke Method"("FPGA VI引用输入"=w65, "错误输入"=w64) -> ("FPGA VI引用输出"=w31:refnum<k20>, "错误输出"=w30:errorcluster)
  n139 = xnode "读取/写入控件"("FPGA VI引用输入"=w59, "错误输入"=w58, "Shutter"=w49, "Start Control"=w49) -> ("FPGA VI引用输出"=w51:refnum<k20>, "错误输出"=w50:errorcluster)
  n140 = xnode "Invoke Method"("FPGA VI引用输入"=w31, "错误输入"=w30) -> ("FPGA VI引用输出"=w55:refnum<k20>, "错误输出"=w54:errorcluster)  [unwired: 1 in]
  n141 = flat-sequence {
    tunnel: w5 -> [_]
    frame #0 {
      n142 = local read "Z"() -> (w360:bool)
      n143 = case shown="假" w360 {
        frame False {
          n144 = property on="Ready" class="Slide (严格)"("Label.Visible"=TRUE ("标签.可见")) -> ()  [unwired: 2 in, 2 out]
          n145 = property on="Z-Stack" class="Bool (严格)"("DisabledEnum"=T4."Enabled" ("禁用")) -> ()  [unwired: 2 in, 2 out]
          n146 = property on="LIVE" class="Bool (严格)"("DisabledEnum"=T4."Enabled" ("禁用")) -> ()  [unwired: 2 in, 2 out]
          n147 = property on="Save" class="Bool (严格)"("DisabledEnum"=T4."Enabled" ("禁用")) -> ()  [unwired: 2 in, 2 out]
          n148 = local write "Ready"(u8 10 ("Process")) -> ()
        }
        frame True {
          n149 = local write "Ready"(u8 6 ("Process")) -> ()
        }
      }
    }
  }
  n150 = while {
    tunnel: w55 -> [w374]
    tunnel: w54 -> [w373]
    tunnel: [w372] -> w19
    tunnel: [w371] -> w6
    tunnel: [w370] -> w52
    tunnel: w51 -> [w370]
    tunnel: [w369] -> w47
    tunnel: w50 -> [w369]
    stop <- w367 stop-if-true
    n151 = xnode "读取/写入控件"("FPGA VI引用输入"=w374, "错误输入"=w373) -> ("FPGA VI引用输出"=w372:refnum<k20>, "错误输出"=w371:errorcluster, "Adapter Module Initialization Done"=w367:bool)
    "Initialization Done" <- w367
    n152 = local write "Ready"(u8 3 ("Process")) -> ()
  }
  n153 = local read "Point/Pixel"() -> (w7:i32)
  n154 = property on="Point/Pixel" class="DigNum (严格)"(error in=w6, "Val(Sgnl)"=w7) -> (error out=w5:errorcluster)  [unwired: 1 in, 1 out]
  n155 = Obtain Queue(name (unnamed)="Display" ("名称（未命名）"), element data type=i16[][] []) -> (queue out=w21:refnum<queue>, error out=w22:errorcluster)  [unwired: 3 in, 1 out]
  n156 = Obtain Queue(name (unnamed)="Save" ("名称（未命名）"), element data type=i16[][] []) -> (queue out=w32:refnum<queue>, error out=w76:errorcluster)  [unwired: 3 in, 1 out]
  n157 = call "IMAQ Create"("Image Name"="Save", "Image Type"=w28) -> ("New Image"=w26:T1)  [unwired: 3 in, 1 out]
  n158 = while {
    tunnel: w32 -> [w384]
    shift-right: [w380] -> _
    shift-left: u16 0 -> [w381]
    shift-right: [w377] -> _
    shift-left: u16 0 -> [w378]
    shift-right: [w375] -> _
    shift-left: w26 -> [w379]
    stop <- w376 stop-if-true
    n159 = Dequeue Element(queue=w384) -> (element=w382:i16[][], error out=w383:errorcluster)  [unwired: 2 in, 2 out]
    n160 = case shown="无错误" w383 {
      tunnel: w382 -> [w388 _]
      tunnel: w381 -> [w400 w461]
      tunnel: [w399 w461] -> w380
      tunnel: w379 -> [w398 w458]
      tunnel: w378 -> [w391 w460]
      tunnel: [w390 w460] -> w377
      tunnel: [FALSE TRUE] -> w376
      tunnel: [w385 w458] -> w375
      frame No Error {
        # "高"
        # "低"
        n161 = local read "Pulse Number"() -> (w387:enum16{"SP", "DP"})
        n162 = call "sub_数组奇数行转置.vi"("Pulse Number"=w387, "Input"=w388) -> ("output"=w386:u16[][])
        n163 = local read "Z-Stack"() -> (w396:bool)
        n164 = Build Array("Save", w396) -> (w395:bool[])
        n165 = Boolean Array To Number(Boolean array=w395) -> (number=w394:u32)
        n166 = case shown="1" w394 {
          tunnel: w400 -> [w403 w420 w438 w456]
          tunnel: [u16 0 w419 w440 u16 0] -> w399
          tunnel: w398 -> [w401 w418 w443 w454]
          tunnel: w386 -> [_ w405 w424 _]
          tunnel: "Path" -> [_ w417 w442 _]
          tunnel: [w403 w416 w436 w456] -> w392
          tunnel: w391 -> [_ _ w437 _]
          tunnel: [u16 0 ("t") u16 0 ("t") w439 u16 0] -> w390
          tunnel: [w401 w406 w425 w454] -> w385
          frame 0, Default {
          }
          frame 1 {
            # "Save"
            n167 = call "IMAQ ArrayToImage"("Image Pixels (U16)"=w405, "Image"=w418) -> ("Image Out"=w408:T1)  [unwired: 8 in, 1 out]
            n168 = Number To Decimal String(number=w420) -> (decimal integer string=w413:string)  [unwired: 1 in]
            n169 = Increment(x=w420) -> (x+1=w416:u16)
            n170 = Concatenate Strings("File Name", w413, ".tif" ("字符串")) -> (w414:string)
            n171 = Greater Or Equal?(x=w416, y="Save Frames") -> (x >= y?=w409:bool)
            n172 = case shown="真" w409 {
              tunnel: [w421 u16 0] -> w419
              tunnel: w416 -> [w421 _]
              frame False {
              }
              frame True {
                n173 = property on="Save" class="Bool (严格)"("Val(Sgnl)"=FALSE ("Save")) -> ()  [unwired: 2 in, 2 out]
              }
            }
            n174 = Build Path(base path=w417, name or relative path=w414) -> (appended path=w411:path)
            n175 = call-poly "IMAQ Write File 2"("File Path"=w411, "Image"=w408) -> ("Image Out (duplicate)"=w406:T1)  [unwired: 8 in, 1 out]
          }
          frame 2 {
            # "Z-Stack"
            n176 = local read "Frames/Slice"() -> (w428:u16)
            n177 = call "IMAQ ArrayToImage"("Image Pixels (U16)"=w424, "Image"=w443) -> ("Image Out"=w430:T1)  [unwired: 8 in, 1 out]
            n178 = Multiply(x=w437, y=w428) -> (x*y=w429:u16)
            n179 = Add(x=w429, y=w438) -> (x+y=w427:u16)
            n180 = Increment(x=w438) -> (x+1=w441:u16)
            n181 = Number To Decimal String(number=w427) -> (decimal integer string=w433:string)  [unwired: 1 in]
            n182 = local read "File Name"() -> (w426:string)
            n183 = Greater Or Equal?(x=w441, y=w428) -> (x >= y?=w435:bool)
            n184 = case shown="真" w435 {
              tunnel: w441 -> [w445 _]
              tunnel: w437 -> [w444 w450]
              tunnel: [w445 u16 0 ("t")] -> w440
              tunnel: [w444 w448] -> w439
              frame False {
              }
              frame True {
                n185 = local read "Slices"() -> (w446:u16)
                n186 = Increment(x=w450) -> (x+1=w447:u16)
                n187 = property on="Z-Stack" class="Bool (严格)"("Val(Sgnl)"=FALSE ("Save")) -> ()  [unwired: 2 in, 2 out]
                n188 = Greater Or Equal?(x=w447, y=w446) -> (x >= y?=w451:bool)
                n189 = Select(t=u16 0, s=w451, f=w447) -> (s? t:f=w448:u16)
              }
            }
            n190 = Concatenate Strings(w426, w433, ".tif" ("字符串")) -> (w434:string)
            n191 = Increment(x=w427) -> (x+1=w436:u16)
            n192 = Build Path(base path=w442, name or relative path=w434) -> (appended path=w431:path)
            n193 = call-poly "IMAQ Write File 2"("File Path"=w431, "Image"=w430) -> ("Image Out (duplicate)"=w425:T1)  [unwired: 8 in, 1 out]
          }
          frame 3 {
          }
        }
        "Save Frames Dis." <- w392
      }
      frame Error {
      }
    }
  }
  n194 = while {
    tunnel: w19 -> [w466]
    tunnel: w5 -> [w465]
    shift-right: [w462] -> _
    shift-left: 0 ("t") -> [w463]
    stop <- w464 stop-if-true
    n195 = event shown="[6] \"16-bit Display Method\", \"Map Max.\", \"Map Min.\", \"Max. Min.\": 值改变" {
      selector: _ -> [_ _ _ _ _ _ _ _ _ _ _ _ _ _]
      dyn-events: _ -> [_ _ _ _ _ _ _ _ _ _ _ _ _ _]
      timeout: _ -> [_ _ _ _ _ _ _ _ _ _ _ _ _ _]
      tunnel: w466 -> [_ w518 _ _ _ _ _ _ _ w638 w646 w696 _ _]
      tunnel: w465 -> [_ w516 _ _ _ _ _ _ _ w637 w645 w695 _ _]
      tunnel: [_ _ _ _ _ _ _ _ _ _ _ _ _ TRUE] -> w464
      tunnel: w463 -> [w467 w505 w522 w537 w553 w574 w584 w592 w623 w636 w643 w693 w733 _]
      tunnel: [w467 w505 w522 w537 w553 w574 w584 w592 w622 w636 w643 w693 w733 u16 0 ("t")] -> w462
      event "XY RIGHT", "XY LEFT", "XY DOWN", "XY UP", "XY Home": Value Change {
        n196 = event-data() -> ()  [unwired: 1 in, 6 out]
        n197 = Build Array("XY Home", "XY UP", "XY DOWN", "XY LEFT", "XY RIGHT") -> (w473:bool[])
        n198 = Boolean Array To Number(Boolean array=w473) -> (number=w474:u32)
        n199 = case shown="16" w474 {
          tunnel: [w478 0.0 w481 w486 w491 w495] -> w476
          tunnel: [w477 0.0 w483 w487 w489 w494] -> w475
          frame 0, Default {
            n200 = local read "X Offset"() -> (w478:dbl)
            n201 = local read "Y Offset"() -> (w477:dbl)
          }
          frame 1 {
            # "Home"
          }
          frame 2 {
            # "UP"
            n202 = local read "Scale Value"() -> (w484:dbl)
            n203 = local read "X Offset"() -> (w481:dbl)
            n204 = local read "Y Offset"() -> (w482:dbl)
            n205 = Add(x=w482, y=w484) -> (x+y=w483:dbl)
          }
          frame 4 {
            # "DOWN"
            n206 = local read "Scale Value"() -> (w488:dbl)
            n207 = local read "Y Offset"() -> (w485:dbl)
            n208 = local read "X Offset"() -> (w486:dbl)
            n209 = Subtract(x=w485, y=w488) -> (x-y=w487:dbl)
          }
          frame 8 {
            # "LEFT"
            n210 = local read "Scale Value"() -> (w492:dbl)
            n211 = local read "X Offset"() -> (w490:dbl)
            n212 = local read "Y Offset"() -> (w489:dbl)
            n213 = Add(x=w490, y=w492) -> (x+y=w491:dbl)
          }
          frame 16 {
            # "RIGHT"
            n214 = local read "Scale Value"() -> (w496:dbl)
            n215 = local read "X Offset"() -> (w493:dbl)
            n216 = local read "Y Offset"() -> (w494:dbl)
            n217 = Subtract(x=w493, y=w496) -> (x-y=w495:dbl)
          }
        }
        n218 = local write "X Offset"(w476) -> ()
        n219 = local write "Y Offset"(w475) -> ()
      }
      event "Nonlinear Acq.", "Point/Pixel", "Microscope", "Wave": Value Change {
        n220 = event-data() -> ()  [unwired: 1 in, 3 out]
        n221 = local read "Wave"() -> (w499:enum16{"Triangle", "Sine", "Ramp"})
        n222 = local read "Acq. Sample Rate"() -> (w515:dbl)
        n223 = local read "X Frequency"() -> (w513:dbl)
        n224 = local read "Fill Fraction"() -> (w514:dbl)
        n225 = local read "Pixel/Line"() -> (w512:u16)
        n226 = Equal?(x=w499, y=enum16{"Triangle", "Sine", "Ramp"}."Sine") -> (x = y?=w497:bool)
        "Nonlinear Acq." <- w497
        n227 = local read "Point/Pixel"() -> (w503:i32)
        n228 = To Double Precision Float(number=w512) -> (double precision float=w511:dbl)
        n229 = call "sub_Sin Acq Point.vi"("Nonlinear Acq."=w497, "Point/Pixel"=w503, "Effecte Pixel/Line"=w511, "Fill Fraction"=w514, "Scanning Speed"=w513, "Sample Rate"=w515) -> ("Total Data Out"=→"Total Data Out":u16, "Init Data Out"=w502:u16[], "Init Data Out FXP"=w501:fxp<+,18,0>[])  [unwired: 3 in]
        "Acq.Point Array" <- w502
        "Init Data Out" <- w502
        n230 = Index Array(array=w502, index=0 ("索引")) -> (element=w506:u16)
        n231 = local write "Acq. Start"(w506) -> ()
        n232 = xnode "Invoke Method"("FPGA VI引用输入"=w518, "错误输入"=w516, "数据"=w501, "超时(ms)"=0) -> ("FPGA VI引用输出"=w510:refnum<k20>, "错误输出"=w509:errorcluster)  [unwired: 1 out]
        n233 = local read "Microscope"() -> (w500:enum16{"Miniature", "Benchtop"})
        n234 = case shown="\"Miniature\", 默认" w500 {
          frame "Miniature", Default {
            n235 = local write "Real Back Period"("Back Period") -> ()
          }
          frame "Benchtop" {
            n236 = local write "Real Back Period"(u16 1 ("Back Period")) -> ()
          }
        }
        n237 = xnode "Invoke Method"("FPGA VI引用输入"=w510, "错误输入"=w509, "数据"=w502, "超时(ms)"=0) -> ()  [unwired: 3 out]
      }
      event "Start Device": Value Change {
        n238 = event-data() -> ()  [unwired: 1 in, 6 out]
        n239 = case shown="假" "Start Device" {
          frame False {
            n240 = flat-sequence {
              frame #0 {
                n241 = local write "Mems Enable"(FALSE ("Mems Enable")) -> ()
                n242 = Wait (ms)(milliseconds to wait=u32 50 ("等待时间（毫秒）")) -> ()  [unwired: 1 out]
              }
              frame #1 {
                n243 = local write "5V"(FALSE ("5V")) -> ()
                n244 = Wait (ms)(milliseconds to wait=u32 50 ("等待时间（毫秒）")) -> ()  [unwired: 1 out]
              }
              frame #2 {
                n245 = local write "Source:Output Enabled"(FALSE ("Source:Output Enabled")) -> ()
                n246 = local write "PMT1 Enable"(FALSE ("PMT1 Enable")) -> ()
              }
            }
          }
          frame True {
            n247 = flat-sequence {
              frame #0 {
                n248 = local write "Source:Output Enabled"(TRUE ("Source:Output Enabled")) -> ()
                n249 = local write "PMT1 Enable"(TRUE ("PMT1 Enable")) -> ()
                n250 = Wait (ms)(milliseconds to wait=u32 50 ("等待时间（毫秒）")) -> ()  [unwired: 1 out]
              }
              frame #1 {
                n251 = local write "5V"(TRUE ("5V")) -> ()
                n252 = Wait (ms)(milliseconds to wait=u32 50 ("等待时间（毫秒）")) -> ()  [unwired: 1 out]
              }
              frame #2 {
                n253 = local write "Mems Enable"(TRUE ("Mems Enable")) -> ()
              }
            }
          }
        }
      }
      event "Add Phase": Value Change {
        n254 = event-data() -> ()  [unwired: 1 in, 6 out]
        n255 = local read "Scan Mode"() -> (w536:enum16{"Normal", "Line Scan", "Random Access"})
        n256 = local read "Phase Shift"() -> (w535:u32)
        n257 = case shown="\"Normal\", 默认" w536 {
          tunnel: w535 -> [w538 w539]
          frame "Random Access" {
            "Random Phase" <- w538
          }
          frame "Normal", Default {
            n258 = local read "Microscope"() -> (w547:enum16{"Miniature", "Benchtop"})
            n259 = case shown="\"Miniature\", 默认" w547 {
              tunnel: [w550 w551] -> w546
              frame "Miniature", Default {
                n260 = local read "Zoom Miniature"() -> (w550:dbl[][])
              }
              frame "Benchtop" {
                n261 = local read "Zoom Standard"() -> (w551:dbl[][])
              }
            }
            n262 = local read "ZOOM"() -> (w545:u16)
            n263 = Decrement(x=w545) -> (x-1=w543:u16)
            n264 = Index Array(array=w546, index (row)=w543) -> (element=w540:dbl[])  [unwired: 1 in]
            n265 = Insert Into Array(array=w540, index=2 ("索引"), new element=w539) -> (w542:dbl[])
            n266 = case shown="0, 默认" w545 {
              frame 0, Default {
                n267 = local read "Phase Shift"() -> (→"User Define Phase":u32)
              }
              frame 1 {
              }
            }
            n268 = Replace Array Subset(array=w546, new element=w542, index (row)=w543) -> (w544:dbl[][])  [unwired: 1 in]
            n269 = case shown="\"Miniature\", 默认" w547 {
              tunnel: w544 -> [w548 w549]
              frame "Miniature", Default {
                n270 = local write "Zoom Miniature"(w548) -> ()
              }
              frame "Benchtop" {
                n271 = local write "Zoom Standard"(w549) -> ()
              }
            }
          }
        }
      }
      event "Scan Mode", "ZOOM": Value Change {
        n272 = event-data() -> ()  [unwired: 1 in, 6 out]
        n273 = local read "Microscope"() -> (w560:enum16{"Miniature", "Benchtop"})
        n274 = case shown="\"Miniature\", 默认" w560 {
          tunnel: [w564 w565] -> w557
          frame "Miniature", Default {
            n275 = local read "Zoom Miniature"() -> (w564:dbl[][])
          }
          frame "Benchtop" {
            n276 = local read "Zoom Standard"() -> (w565:dbl[][])
          }
        }
        n277 = local read "ZOOM"() -> (w556:u16)
        n278 = case shown="0, 默认" w556 {
          selector: w556 -> [_ w569]
          tunnel: w557 -> [_ w570]
          tunnel: [w566 w568] -> w559
          frame 0, Default {
            n279 = local read "User Define Phase"() -> (w566:u32)
          }
          frame 1..10 {
            n280 = Decrement(x=w569) -> (x-1=w572:u16)
            n281 = Index Array(array=w570, index (row)=w572) -> (element=w573:dbl[])  [unwired: 1 in]
            n282 = Index Array(array=w573, index=2 ("索引")) -> (element=w567:dbl)
            n283 = To Unsigned Long Integer(number=w567) -> (unsigned 32bit integer=w568:u32)
          }
        }
        n284 = local read "Random Phase"() -> (w558:u32)
        n285 = local read "Scan Mode"() -> (w555:enum16{"Normal", "Line Scan", "Random Access"})
        n286 = case shown="\"Normal\", 默认" w555 {
          tunnel: w559 -> [w561 w562 _]
          tunnel: w558 -> [_ _ w563]
          tunnel: [w561 w562 w563] -> w554
          frame "Normal", Default {
          }
          frame "Line Scan" {
          }
          frame "Random Access" {
          }
        }
        n287 = local write "Phase Shift"(w554) -> ()
      }
      event "Set Large Scale", "Set Small Scale", "Scale": Value Change {
        n288 = event-data() -> ()  [unwired: 1 in, 6 out]
        n289 = Select(t="Set Large Scale", s="Scale", f="Set Small Scale") -> (s? t:f=→"Scale Value":dbl)
      }
      event "16-bit Display Method", "Map Max.", "Map Min.", "Max. Min.": Value Change {
        w580 = 32768 ("y")
        n290 = event-data() -> ()  [unwired: 1 in, 6 out]
        n291 = local read "16-bit Display Method"() -> (w585:u32)
        n292 = Unbundle("Max. Min.") -> (w582:i32, w581:i32)
        n293 = case shown="14" w585 {
          frame 0, Default {
          }
          frame 14 {
            n294 = To Double Precision Float(number="Map Max.") -> (double precision float=w589:dbl)
            n295 = To Double Precision Float(number="Map Min.") -> (double precision float=w588:dbl)
            n296 = property on="Max. Min." class="Slide (严格)"("Scale.Maximum"=w589, "Scale.Minimum"=w588) -> ()  [unwired: 2 in, 2 out]
          }
        }
        n297 = Add(x=w582, y=w580) -> (x+y=w583:i32)
        n298 = Add(x=w581, y=w580) -> (x+y=w579:i32)
        n299 = property on="Image" class="ImageControl"("16-bit Display Conversion Method"="16-bit Display Method", "16-bit Display Maximum Value"=w583, "16-bit Display Minimum Value"=w579) -> ()  [unwired: 2 in, 2 out]
      }
      event "Image": Mouse Up {
        n300 = event-data() -> ()  [unwired: 1 in, 8 out]
        n301 = disable-structure shown="禁用" {
          frame Disabled {
            n302 = local read "Microscope"() -> (w596:enum16{"Miniature", "Benchtop"})
            n303 = case shown="\"Benchtop\"" w596 {
              tunnel: [w606 w607] -> w597
              frame "Miniature", Default {
                n304 = local read "Zoom Miniature"() -> (w606:dbl[][])
              }
              frame "Benchtop" {
                n305 = local read "Zoom Standard"() -> (w607:dbl[][])
              }
            }
            n306 = local read "ZOOM"() -> (w595:u16)
            n307 = case shown="0, 默认" w595 {
              selector: w595 -> [_ w612]
              tunnel: [w608 w610] -> w593
              tunnel: [w609 w611] -> w594
              tunnel: w597 -> [_ w613]
              frame 0, Default {
                n308 = local read "X Amplitude"() -> (w609:dbl)
                n309 = local read "Y Amplitude"() -> (w608:dbl)
              }
              frame 1..10 {
                n310 = Decrement(x=w612) -> (x-1=w616:u16)
                n311 = Index Array(array=w613, index (row)=w616) -> (element=w617:dbl[])  [unwired: 1 in]
                n312 = Index Array(array=w617, index #1=0 ("索引"), index #2=1 ("索引")) -> (element #1=w611:dbl, element #2=w610:dbl)  [unwired: 1 in, 1 out]
              }
            }
            n313 = property on="Image" class="ImageControl"() -> ("ROI"=w605:T5)  [unwired: 2 in, 2 out]
            n314 = local read "Pixel/Line"() -> (w602:u16)
            n315 = local read "Line"() -> (w601:u32)
            n316 = Unbundle By Name(w605) -> ("Global Rectangle"=w604:i32[])
            n317 = call "sub_new x y amplitude.vi"("Global Rectangle"=w604, "Line"=w601, "Pixel/Line"=w602, "y amp."=w593, "x amp."=w594) -> ("y offset new"=→"y offset new":i16, "x offset new"=→"x offset new":i16, "y amp. new"=→"y amp. new":dbl, "x amp. new"=→"x amp. new":dbl)  [unwired: 3 in]
          }
          frame Enabled {
          }
        }
      }
      event "Add Random Access", "Clear Array": Value Change {
        n318 = event-data() -> ()  [unwired: 1 in, 6 out]
        n319 = case shown="真" "Add Random Access" {
          tunnel: w623 -> [w626 w630]
          tunnel: [w626 w631] -> w620
          frame False {
          }
          frame True {
            n320 = local read "x amp. new"() -> (w635:dbl)
            n321 = local read "y amp. new"() -> (w634:dbl)
            n322 = local read "x offset new"() -> (w633:i16)
            n323 = local read "y offset new"() -> (w632:i16)
            n324 = call "sub_new amplitude to array.vi"("Index Row"=w630, "All Random Array In"="All Random Array", "y offset new"=w632, "x offset new"=w633, "y amp. new"=w634, "x amp. new"=w635) -> ("All Random Array Out"=w628:fxp<+/-,32,16>[][])  [unwired: 4 in, 1 out]
            n325 = Increment(x=w630) -> (x+1=w631:i32)
            n326 = local write "All Random Array"(w628) -> ()
            n327 = call "sub_2D Array to 1D.vi"("2D Array"=w628) -> ("Random 1D Array"=w627:fxp<+/-,32,16>[])
            n328 = local write "Random 1D Array"(w627) -> ()
          }
        }
        n329 = case shown="真" "Clear Array" {
          frame False {
          }
          frame True {
            n330 = local write "Random 1D Array"(fxp<+/-,32,16>[] [0.0, 0.0, 0.0, 0.0, 0.0, 0.0, 0.0, 0.0, 0.0, 0.0, 0.0, 0.0, 0.0, 0.0, 0.0, 0.0, 0.0, 0.0, 0.0, 0.0, 0.0, 0.0, 0.0, 0.0, 0.0, 0.0, 0.0, 0.0, 0.0, 0.0, 0.0, 0.0, 0.0, 0.0, 0.0, 0.0, 0.0, 0.0, 0.0, 0.0, 0.0, 0.0, 0.0, 0.0, 0.0, 0.0, 0.0, 0.0, 0.0, 0.0, 0.0, 0.0, 0.0, 0.0, 0.0, 0.0, 0.0, 0.0, 0.0, 0.0, 0.0, 0.0, 0.0, 0.0, 0.0, 0.0, 0.0, 0.0, 0.0, 0.0, 0.0, 0.0, 0.0, 0.0, 0.0, 0.0, 0.0, 0.0, 0.0, 0.0, 0.0, 0.0, 0.0, 0.0, 0.0, 0.0, 0.0, 0.0, 0.0, 0.0, 0.0, 0.0, 0.0, 0.0, 0.0, 0.0, 0.0, 0.0, 0.0, 0.0, 0.0, 0.0, 0.0, 0.0, 0.0, 0.0, 0.0, 0.0, 0.0, 0.0, 0.0, 0.0, 0.0, 0.0, 0.0, 0.0, 0.0, 0.0, 0.0, 0.0, 0.0, 0.0, 0.0, 0.0, 0.0, 0.0, 0.0, 0.0, 0.0, 0.0, 0.0, 0.0, 0.0, 0.0, 0.0, 0.0, 0.0, 0.0, 0.0, 0.0, 0.0, 0.0, 0.0, 0.0, 0.0, 0.0, 0.0, 0.0, 0.0, 0.0, 0.0, 0.0, 0.0, 0.0, 0.0, 0.0, 0.0, 0.0, 0.0, 0.0, 0.0, 0.0, 0.0, 0.0, 0.0, 0.0, 0.0, 0.0, 0.0, 0.0, 0.0, 0.0, 0.0, 0.0, 0.0, 0.0, 0.0, 0.0, 0.0, 0.0, 0.0, 0.0, 0.0, 0.0, 0.0, 0.0, 0.0, 0.0, 0.0, 0.0, 0.0, 0.0, 0.0, 0.0, 0.0, 0.0, 0.0, 0.0, 0.0, 0.0] ("Random 1D Array")) -> ()
            n331 = local write "All Random Array"(fxp<+/-,32,16>[][] [] ("All Random Array")) -> ()
          }
        }
        n332 = Select(t=0, s="Clear Array", f=w620) -> (s? t:f=w622:i32)
      }
      event "Apply": Value Change {
        n333 = event-data() -> ()  [unwired: 1 in, 6 out]
        n334 = xnode "读取/写入控件"("FPGA VI引用输入"=w638, "错误输入"=w637, "Adapter Module User Command"="Adapter Module User Command", "Adapter Module User Data 0"="Adapter Module User Data 0", "Adapter Module User Data 1"="Adapter Module User Data 1", "Adapter Module Do User Command Commit"="Apply") -> ()  [unwired: 2 out]
      }
      event "Gain": Value Change {
        n335 = event-data() -> ()  [unwired: 1 in, 6 out]
        n336 = local read "Microscope"() -> (w644:enum16{"Miniature", "Benchtop"})
        n337 = case shown="\"0dB\", 默认" "Gain" {
          tunnel: w646 -> [w650 w665 w680]
          tunnel: w645 -> [w649 w664 w679]
          tunnel: w644 -> [w648 w663 w678]
          frame "0dB", Default {
            n338 = case shown="\"Miniature\", 默认" w648 {
              tunnel: w650 -> [w656 w658]
              tunnel: w649 -> [w655 w657]
              frame "Miniature", Default {
                n339 = xnode "读取/写入控件"("FPGA VI引用输入"=w656, "错误输入"=w655, "Adapter Module User Command"=u8 2, "Adapter Module User Data 0"=u8 0, "Adapter Module User Data 1"=u8 0, "Adapter Module Do User Command Commit"=TRUE) -> ()  [unwired: 2 out]
              }
              frame "Benchtop" {
                n340 = xnode "读取/写入控件"("FPGA VI引用输入"=w658, "错误输入"=w657, "Adapter Module User Command"=u8 2, "Adapter Module User Data 0"=u8 1, "Adapter Module User Data 1"=u8 0, "Adapter Module Do User Command Commit"=TRUE) -> ()  [unwired: 2 out]
              }
            }
          }
          frame "6dB" {
            n341 = case shown="\"Benchtop\"" w663 {
              tunnel: w665 -> [w671 w673]
              tunnel: w664 -> [w670 w672]
              frame "Miniature", Default {
                n342 = xnode "读取/写入控件"("FPGA VI引用输入"=w671, "错误输入"=w670, "Adapter Module User Command"=u8 2, "Adapter Module User Data 0"=u8 0, "Adapter Module User Data 1"=u8 1, "Adapter Module Do User Command Commit"=TRUE) -> ()  [unwired: 2 out]
              }
              frame "Benchtop" {
                n343 = xnode "读取/写入控件"("FPGA VI引用输入"=w673, "错误输入"=w672, "Adapter Module User Command"=u8 2, "Adapter Module User Data 0"=u8 1, "Adapter Module User Data 1"=u8 1, "Adapter Module Do User Command Commit"=TRUE) -> ()  [unwired: 2 out]
              }
            }
          }
          frame "12dB" {
            n344 = case shown="\"Miniature\", 默认" w678 {
              tunnel: w680 -> [w682 w692]
              tunnel: w679 -> [w681 w691]
              frame "Miniature", Default {
                n345 = xnode "读取/写入控件"("FPGA VI引用输入"=w682, "错误输入"=w681, "Adapter Module User Command"=u8 2, "Adapter Module User Data 0"=u8 0, "Adapter Module User Data 1"=u8 2, "Adapter Module Do User Command Commit"=TRUE) -> ()  [unwired: 2 out]
              }
              frame "Benchtop" {
                n346 = xnode "读取/写入控件"("FPGA VI引用输入"=w692, "错误输入"=w691, "Adapter Module User Command"=u8 2, "Adapter Module User Data 0"=u8 1, "Adapter Module User Data 1"=u8 2, "Adapter Module Do User Command Commit"=TRUE) -> ()  [unwired: 2 out]
              }
            }
          }
        }
      }
      event "Coulple": Value Change {
        n347 = event-data() -> ()  [unwired: 1 in, 6 out]
        n348 = local read "Microscope"() -> (w694:enum16{"Miniature", "Benchtop"})
        n349 = case shown="\"AC\", 默认" "Coulple" {
          tunnel: w696 -> [w700 w715]
          tunnel: w695 -> [w699 w714]
          tunnel: w694 -> [w698 w713]
          frame "AC", Default {
            n350 = case shown="\"Benchtop\"" w698 {
              tunnel: w700 -> [w702 w708]
              tunnel: w699 -> [w701 w707]
              frame "Miniature", Default {
                n351 = xnode "读取/写入控件"("FPGA VI引用输入"=w702, "错误输入"=w701, "Adapter Module User Command"=u8 3, "Adapter Module User Data 0"=u8 0, "Adapter Module User Data 1"=u8 0, "Adapter Module Do User Command Commit"=TRUE) -> ()  [unwired: 2 out]
              }
              frame "Benchtop" {
                n352 = xnode "读取/写入控件"("FPGA VI引用输入"=w708, "错误输入"=w707, "Adapter Module User Command"=u8 3, "Adapter Module User Data 0"=u8 1, "Adapter Module User Data 1"=u8 0, "Adapter Module Do User Command Commit"=TRUE) -> ()  [unwired: 2 out]
              }
            }
          }
          frame "DC" {
            n353 = case shown="\"Benchtop\"" w713 {
              tunnel: w715 -> [w717 w723]
              tunnel: w714 -> [w716 w722]
              frame "Miniature", Default {
                n354 = xnode "读取/写入控件"("FPGA VI引用输入"=w717, "错误输入"=w716, "Adapter Module User Command"=u8 3, "Adapter Module User Data 0"=u8 0, "Adapter Module User Data 1"=u8 1, "Adapter Module Do User Command Commit"=TRUE) -> ()  [unwired: 2 out]
              }
              frame "Benchtop" {
                n355 = xnode "读取/写入控件"("FPGA VI引用输入"=w723, "错误输入"=w722, "Adapter Module User Command"=u8 3, "Adapter Module User Data 0"=u8 1, "Adapter Module User Data 1"=u8 1, "Adapter Module Do User Command Commit"=TRUE) -> ()  [unwired: 2 out]
              }
            }
          }
        }
      }
      event "Frames/Slice", "Slices": Value Change {
        n356 = event-data() -> ()  [unwired: 1 in, 6 out]
        n357 = local read "Start Dis."() -> (w731:sgl)
        n358 = local read "End Dis."() -> (w732:sgl)
        n359 = Subtract(x=w732, y=w731) -> (x-y=w730:sgl)
        n360 = Divide(x=w730, y="Slices") -> (x/y=w728:sgl)
        n361 = local write "Interval Dis."(w728) -> ()
      }
      event "Stop": Value Change {
        n362 = event-data() -> ()  [unwired: 1 in, 6 out]
      }
    }
  }
  n363 = while {
    tunnel: [w741] -> w57
    tunnel: [w740] -> w56
    tunnel: w52 -> [w739]
    tunnel: w47 -> [w738]
    stop <- w736 stop-if-true
    n364 = event shown="[0] 超时" {
      selector: _ -> [_ _]
      dyn-events: _ -> [_ _]
      timeout: 1 -> [_ _]
      tunnel: [w778 w860] -> w741
      tunnel: [w777 w859] -> w740
      tunnel: w739 -> [w780 w862]
      tunnel: w738 -> [w779 w861]
      tunnel: [_ TRUE ("FPGA Stop")] -> w736
      event Timeout {
        n365 = event-data() -> ()  [unwired: 1 in, 3 out]
        n366 = local read "Pulse Number"() -> (w760:enum16{"SP", "DP"})
        n367 = local read "Acq. Sample Rate"() -> (w750:dbl)
        n368 = Equal?(x=w760, y=enum16{"SP", "DP"}."SP") -> (x = y?=w758:bool)
        n369 = local read "Microscope"() -> (w801:enum16{"Miniature", "Benchtop"})
        n370 = case shown="\"Benchtop\"" w801 {
          tunnel: ["Zoom Miniature" "Zoom Standard"] -> w800
          frame "Miniature", Default {
          }
          frame "Benchtop" {
          }
        }
        n371 = local read "Total Data Out"() -> (w754:u16)
        n372 = Select(t=1.0, s=w758, f=2.0 ("t")) -> (s? t:f=w757:dbl)
        n373 = local read "Wave"() -> (w761:enum16{"Triangle", "Sine", "Ramp"})
        n374 = call "sub_MEMS Value to Frequency.vi"("MEMS FAST"="MEMS FAST") -> ("Ticks"=w811:u32)  [unwired: 10 in]
        n375 = call "sub_MEMS Value to Frequency.vi"("MEMS FAST"="MEMS SLOW") -> ("Ticks"=w812:u32)  [unwired: 10 in]
        n376 = case shown="0, 默认" "ZOOM" {
          selector: "ZOOM" -> [_ w852]
          tunnel: ["Y Amplitude" w850] -> w798
          tunnel: ["X Amplitude" w851] -> w803
          tunnel: w800 -> [_ w853]
          frame 0, Default {
          }
          frame 1..10 {
            n377 = Decrement(x=w852) -> (x-1=w856:u16)
            n378 = Index Array(array=w853, index (row)=w856) -> (element=w857:dbl[])  [unwired: 1 in]
            n379 = Index Array(array=w857, index #1=0 ("索引"), index #2=1 ("索引")) -> (element #1=w851:dbl, element #2=w850:dbl)  [unwired: 1 in, 1 out]
          }
        }
        n380 = local read "Line"() -> (w816:u32)
        n381 = Multiply(x="X Frequency", y=w757) -> (x*y=w818:dbl)
        n382 = Divide(x=w818, y=w816) -> (x/y=→"Frame Rate":dbl)
        n383 = call "sub_HOSTTOFPGA Voltage.vi"("Input"="Y Offset") -> ("Output"=w788:i16)
        n384 = call "sub_HOSTTOFPGA Voltage.vi"("Input"="X Offset") -> ("Output"=w753:i16)
        n385 = call "sub_HOSTTOFPGA Voltage.vi"("Input"="Laser Intensity") -> ("Output"=w785:i16)
        n386 = call "sub_HOSTTOFPGA Voltage.vi"("Input"="PMT1 Sensitivity") -> ("Output"=w792:i16)
        n387 = call "sub_HOSTTOFPGA Voltage.vi"("Input"="PMT2 Sensitivity") -> ("Output"=w771:i16)
        n388 = To Word Integer(number=w792) -> (16bit integer=w839:i16)
        n389 = case shown="\"Line Scan\"" "Scan Mode" {
          tunnel: [w843 0.0 ("数值输入控件") w845] -> w804
          tunnel: w798 -> [w843 _ w845]
          frame "Normal", Default {
          }
          frame "Line Scan" {
          }
          frame "Random Access" {
          }
        }
        n390 = To Word Integer(number=w771) -> (16bit integer=w769:i16)
        n391 = To Word Integer(number=w785) -> (16bit integer=w786:i16)
        n392 = local read "Acq. Sample Rate"() -> (w751:dbl)
        n393 = call "sub_XY Amplitude Regular.vi"("Y Amplitude"=w804, "X Amplitude"=w803) -> ("Y Amplitude Out"=w806:fxp<+,16,0>, "X Amplitude Out"=w805:fxp<+,16,0>)  [unwired: 8 in]
        n394 = local read "Wave"() -> (w765:enum16{"Triangle", "Sine", "Ramp"})
        n395 = case shown="\"SP\"" "Pulse Number" {
          tunnel: [enum16{"Single Pulse", "Two Pulse"}."Two Pulse" ("Pulse Number") enum16{"Single Pulse", "Two Pulse"}."Single Pulse" ("Pulse Number")] -> w764
          frame "DP" {
          }
          frame "SP" {
          }
        }
        n396 = call "sub_calculate value.vi"("Pixel/Line"="Pixel/Line", "Fill Fraction"="Fill Fraction", "Wave"=w765, "X Frequency"="X Frequency", "Acq. Sample Rate"=w751) -> ("Pixel Dwell"=→"Pixel Dwell":dbl, "Point/Pixel"=w748:i32)  [unwired: 5 in]
        "Point/Pixel" <- w748
        n397 = feedback #1() -> (w743:u32)  [unwired: 1 in]
        n398 = call "sub_calculate xyfrequency.vi"("Total Data Out"=w754, "Line"="Line", "Actual Output Ticks"=w743, "Actual DDS Ticks"=w743, "X Frequency"="X Frequency", "Acq. Sample Rate"=w750, "Fill Fraction"="Fill Fraction", "Back Period"="Real Back Period", "Wave"=w761) -> ("Actual DDS Sample Freq"=w784:u32, "Y Ramp Step"=w752:fxp<+/-,24,16>, "Line Out"=w782:u32, "Acq. Latch Time"=w787:u32, "Y Step"=w781:fxp<+/-,24,16>)  [unwired: 2 in]
        "Actual DDS Sample Freq" <- w784
        n399 = xnode "读取/写入控件"("FPGA VI引用输入"=w780, "错误输入"=w779, "Phase Increse"=w784, "Y Ramp Step"=w752, "Line"=w782, "Y Step"=w781, "Latch Time"=w787, "Back Period"="Real Back Period", "Laser Intensity"=w786, "X Offset"=w753, "Y Offset"=w788, "MEMS FAST"=w811, "MEMS SLOW"=w812, "PMT Sensitivity"=w839, "PMT2 Sensitivity"=w769, "X Amplitude"=w805, "Y Amplitude"=w806, "Syn. Latch Time"=u32 4 ("Latch Time"), "Pulse Number"=w764) -> ("FPGA VI引用输出"=w789:refnum<k20>, "错误输出"=w790:errorcluster, "Actual DDS Ticks"=w783:u32)
        "Actual DDS Ticks" <- w783
        n400 = feedback-in #1(w783) -> ()
        n401 = call "sub_HOSTTOFPGA Voltage.vi"("Input"="Stimulate Value") -> ("Output"=w819:i16)
        n402 = Increment(x="Frames Befor Stimulate") -> (x+1=w824:u32)
        n403 = Multiply(x="Stimulate Time", y=u32 500) -> (x*y=w826:u32)
        n404 = To Word Integer(number=w819) -> (16bit integer=w828:i16)
        n405 = xnode "读取/写入控件"("FPGA VI引用输入"=w789, "错误输入"=w790, "DDS Ticks"="DDS Ticks", "Phase Shift"="Phase Shift", "Microscope"="Microscope", "Point"="Point", "PMT1 Enable"="PMT1 Enable", "PMT2 Enable"="PMT2 Switch", "Frames Befor Stimulate"=w824, "Stimulate Interval"="Stimulate Interval", "Stimulate Time"=w826, "Stimulate Enable"="Stimulate Enable", "Vision Stimulate Value"=w828, "Wave"="Wave", "MEMS Enable"="Mems Enable", "OUTPUT Value Ticks"="OUTPUT Value Ticks", "PMT Shutter Pow."="PMT Shutter Pow.") -> ("FPGA VI引用输出"=w778:refnum<k20>, "错误输出"=w777:errorcluster, "Actual Laser Intensity"=w808:i16, "Frame Number"=w837:u32, "Stmulate Interval Dis."=→"Stimulate Time Dis.":u32, "Shock Detection"=→"Overload Dis.":bool, "Actual OUTPUT Value Ticks"=→"Actual OUTPUT Value Ticks":u32)
        n406 = call "值已改变(I32).vi"("输入数据"=w748) -> ("已更改"=w749:bool)  [unwired: 3 in]
        n407 = case shown="真" w749 {
          tunnel: w748 -> [_ w840]
          frame False {
          }
          frame True {
            n408 = property on="Point/Pixel" class="DigNum (严格)"("Val(Sgnl)"=w840) -> ()  [unwired: 2 in, 2 out]
          }
        }
        n409 = local read "Stimulate Interval"() -> (w836:u32)
        n410 = call "sub_FPGATOHOST Voltage.vi"("Input"=w808) -> ("Output"=→"Actual Laser Intensity":dbl)
        n411 = local read "Frame Rate"() -> (w835:dbl)
        n412 = Decrement(x=w837) -> (x-1=w832:u32)
        "Frame Number" <- w832
        n413 = To Double Precision Float(number=w832) -> (double precision float=w831:dbl)
        n414 = Reciprocal(x=w835) -> (1/x=w830:dbl)
        n415 = To Double Precision Float(number=w836) -> (double precision float=w833:dbl)
        n416 = Multiply(x=w831, y=w830) -> (x*y=→"Frame Befor Time":dbl)
        n417 = Multiply(x=w833, y=w830) -> (x*y=→"Stimulate Interval Time":dbl)
      }
      event "Stop": Value Change {
        n418 = event-data() -> ()  [unwired: 1 in, 3 out]
        n419 = xnode "读取/写入控件"("FPGA VI引用输入"=w862, "错误输入"=w861, "FPGA Stop"=TRUE) -> ("FPGA VI引用输出"=w864:refnum<k20>, "错误输出"=w865:errorcluster)
        n420 = xnode "Invoke Method"("FPGA VI引用输入"=w864, "错误输入"=w865) -> ("FPGA VI引用输出"=w860:refnum<k20>, "错误输出"=w859:errorcluster)
      }
    }
  }
  n421 = while {
    tunnel: w19 -> [w881]
    tunnel: w5 -> [w880]
    tunnel: [w879] -> w72
    tunnel: [w878] -> w71
    tunnel: w32 -> [w877]
    tunnel: w76 -> [w876]
    tunnel: [w875] -> w73
    tunnel: w52 -> [w872]
    tunnel: w47 -> [w871]
    border: u32 0 -> [_]
    shift-right: [w869] -> _
    shift-left: u16 0 -> [w870]
    tunnel: w21 -> [w868]
    tunnel: w22 -> [w867]
    tunnel: [w866] -> w20
    stop <- w874 stop-if-true
    # "Z-stack"
    n422 = event shown="[0] 超时" {
      selector: _ -> [_ _ _ _ _]
      dyn-events: _ -> [_ _ _ _ _]
      timeout: 1 -> [_ _ _ _ _]
      tunnel: w881 -> [w897 w998 w1146 w1286 w1313]
      tunnel: w880 -> [w896 w997 w1145 w1285 w1312]
      tunnel: [w903 w996 w1144 w1283 w1315] -> w879
      tunnel: [w899 w990 w1138 w1282 w1314] -> w878
      tunnel: w877 -> [w902 _ _ _ _]
      tunnel: w876 -> [w901 w995 w1143 w1280 w1310]
      tunnel: [w900 w995 w1143 w1280 w1310] -> w875
      tunnel: [_ _ _ _ TRUE] -> w874
      tunnel: w872 -> [_ w994 w1142 _ _]
      tunnel: w871 -> [_ w993 w1141 _ _]
      tunnel: w870 -> [w898 _ w1136 w1281 w1309]
      tunnel: [w898 u16 0 w1135 w1281 w1309] -> w869
      tunnel: w868 -> [w894 _ _ _ _]
      tunnel: w867 -> [w893 w987 w1134 w1273 w1308]
      tunnel: [w892 w987 w1134 w1273 w1308] -> w866
      event Timeout {
        n423 = event-data() -> ()  [unwired: 1 in, 3 out]
        n424 = local read "Microscope"() -> (w883:enum16{"Miniature", "Benchtop"})
        n425 = local read "Pixel/Line"() -> (w886:u16)
        n426 = local read "Line"() -> (w882:u32)
        n427 = Reciprocal(x="Acq. Start") -> (1/x=w890:dbl)
        n428 = To Fixed-Point(fixed-point type=fxp<+,18,0> 0.0, number=w890) -> (fixed-point=w889:fxp<+,18,0>)
        n429 = case shown="真" "Focus Flag" {
          tunnel: w897 -> [w911 w929]
          tunnel: w896 -> [w910 w928]
          tunnel: [w909 w935] -> w903
          tunnel: w902 -> [_ w938]
          tunnel: w901 -> [w917 w937]
          tunnel: [w917 w936] -> w900
          tunnel: [w908 w934] -> w899
          tunnel: w886 -> [_ w930]
          tunnel: w882 -> [_ w921]
          tunnel: w894 -> [_ w933]
          tunnel: w893 -> [w906 w932]
          tunnel: [w906 w931] -> w892
          frame False {
            (unwired) u32 0 ("剩余元素")
            n430 = xnode "Invoke Method"("FPGA VI引用输入"=w911, "错误输入"=w910, "元素数量"=u32 0, "超时(ms)"=0) -> ("FPGA VI引用输出"=w913:refnum<k20>, "错误输出"=w914:errorcluster, "剩余元素"=w905:u32)  [unwired: 1 out]
            n431 = Not Equal To 0?(x=w905) -> (x != 0?=w907:bool)
            n432 = local write "Rolling Queue Flag"(TRUE ("Rolling Queue Flag")) -> ()
            n433 = xnode "Invoke Method"("FPGA VI引用输入"=w913, "错误输入"=w914, "元素数量"=w905, "超时(ms)"=0) -> ("FPGA VI引用输出"=w909:refnum<k20>, "错误输出"=w908:errorcluster)  [unwired: 2 out]
            n434 = case shown="真" w907 {
              frame False {
              }
              frame True {
                n435 = feedback #2() -> (w918:u32)
                n436 = Increment(x=w918) -> (x+1=w919:u32)
                "Test Point" <- w919
                n437 = feedback-in #2(w919) -> ()
              }
            }
          }
          frame True {
            n438 = xnode "Invoke Method"("FPGA VI引用输入"=w929, "错误输入"=w928, "元素数量"=u32 0, "超时(ms)"=0) -> ("FPGA VI引用输出"=w927:refnum<k20>, "错误输出"=w926:errorcluster, "剩余元素"=w925:u32)  [unwired: 1 out]
            n439 = Multiply(x=w930, y=w921) -> (x*y=w920:u32)
            n440 = Greater Or Equal?(x=w925, y=w920) -> (x >= y?=w924:bool)
            n441 = case shown="真" w924 {
              tunnel: w938 -> [_ w968]
              tunnel: w937 -> [w940 w967]
              tunnel: [w940 w966] -> w936
              tunnel: [w942 w965] -> w935
              tunnel: [w941 w964] -> w934
              tunnel: w926 -> [w941 w963]
              tunnel: w927 -> [w942 w962]
              tunnel: w921 -> [_ w956]
              tunnel: w930 -> [_ w955]
              tunnel: w933 -> [_ w961]
              tunnel: w932 -> [w939 w960]
              tunnel: [w939 w959] -> w931
              tunnel: w920 -> [_ w958]
              frame False {
              }
              frame True {
                n442 = xnode "Invoke Method"("FPGA VI引用输入"=w962, "错误输入"=w963, "元素数量"=w958, "超时(ms)"=0) -> ("FPGA VI引用输出"=w965:refnum<k20>, "错误输出"=w964:errorcluster, "数据"=w954:fxp<+,33,17>[])  [unwired: 1 out]
                n443 = To Unsigned Word Integer(number=w954) -> (unsigned 16bit integer=w943:u16[])
                n444 = local read "Read offset"() -> (w946:bool)
                n445 = local read "Offset value"() -> (w947:i16)
                n446 = Reshape Array(w943, w956, w955) -> (w949:u16[][])
                n447 = Select(t=i16 0, s=w946, f=w947) -> (s? t:f=w944:i16)
                n448 = Add(x=w949, y=w944) -> (x+y=w948:u16[][])
                n449 = local read "Read offset"() -> (w952:bool)
                n450 = local read "Z-Stack"() -> (w950:bool)
                n451 = local read "Save"() -> (w951:bool)
                n452 = Enqueue Element(queue=w961, element=w948, error in (no error)=w960) -> (error out=w959:errorcluster)  [unwired: 1 in, 2 out]
                n453 = disable-structure shown="禁用" {
                  frame Disabled {
                    # "转换成I16"
                    n454 = To Unsigned Word Integer() -> (unsigned 16bit integer=w970:u16)  [unwired: 1 in]
                    n455 = Exclusive Or(1:w970, 2:u16 32768 ("x")) -> (0:w971:u16)
                    n456 = To Word Integer(number=w971) -> ()  [unwired: 1 out]
                  }
                  frame Enabled {
                  }
                }
                n457 = Compound Arithmetic op=OR ("复合运算")(w952, w950, w951) -> (w953:bool)
                n458 = case shown="真" w953 {
                  tunnel: w968 -> [_ w976]
                  tunnel: w967 -> [w972 w975]
                  tunnel: [w972 w974] -> w966
                  tunnel: w948 -> [_ w973]
                  frame False {
                  }
                  frame True {
                    n459 = Enqueue Element(queue=w976, element=w973, error in (no error)=w975) -> (error out=w974:errorcluster)  [unwired: 1 in, 2 out]
                  }
                }
              }
            }
          }
        }
        n460 = xnode "读取/写入控件"("FPGA VI引用输入"=w897, "Pixel/Line"=w886, "Line"=w882, "Microscope"=w883, "Acq.Start FXP"=w889, "Acq.Start"="Acq. Start", "Divide"="Divide") -> ("Acq. Point Dis."=→"Acq. Point Dis.":u16)  [unwired: 1 in, 2 out]
        n461 = call "sub_Acquisition Rate.vi"("Divide"="Divide") -> ("采样率"=→"Acq. Sample Rate":dbl)
      }
      event "LIVE", "Save": Value Change {
        (unwired) 0
        (unwired) u16 0
        # "4"
        # "2"
        # "1"
        # "高"
        # "低"
        n462 = event-data() -> ()  [unwired: 1 in, 6 out]
        n463 = local read "Save"() -> (w982:bool)
        n464 = local read "Read offset"() -> (w980:bool)
        n465 = global write "Save picture camera.vi" "Save Picture Camera"(w982) -> ()
        n466 = Build Array("LIVE", w982) -> (w983:bool[])
        n467 = Build Array(w982, "LIVE") -> (w989:bool[])
        n468 = Boolean Array To Number(Boolean array=w983) -> (number=w981:u32)
        n469 = Select(t=FALSE ("Shutter"), s=w980, f=TRUE ("Shutter")) -> (s? t:f=w977:bool)
        n470 = Boolean Array To Number(Boolean array=w989) -> (number=w988:u32)
        n471 = case shown="0, 默认" w988 {
          frame 1 {
            # "SAVE 1"
            # "LIVE 0"
            n472 = property on="LIVE" class="Bool (严格)"("DisabledEnum"=T4."Disabled and Grayed Out" ("禁用")) -> ()  [unwired: 2 in, 2 out]
            n473 = property on="Z-Stack" class="Bool (严格)"("DisabledEnum"=T4."Disabled and Grayed Out" ("禁用")) -> ()  [unwired: 2 in, 2 out]
          }
          frame 2 {
            # "SAVE 0"
            # "LIVE 1"
            n474 = property on="Save" class="Bool (严格)"("DisabledEnum"=T4."Disabled and Grayed Out" ("禁用")) -> ()  [unwired: 2 in, 2 out]
            n475 = property on="Z-Stack" class="Bool (严格)"("DisabledEnum"=T4."Disabled and Grayed Out" ("禁用")) -> ()  [unwired: 2 in, 2 out]
          }
          frame 0, Default {
            # "SAVE 0"
            # "LIVE 0"
            n476 = property on="Save" class="Bool (严格)"("DisabledEnum"=T4."Enabled" ("禁用")) -> ()  [unwired: 2 in, 2 out]
            n477 = property on="LIVE" class="Bool (严格)"("DisabledEnum"=T4."Enabled" ("禁用")) -> ()  [unwired: 2 in, 2 out]
            n478 = property on="Z-Stack" class="Bool (严格)"("DisabledEnum"=T4."Enabled" ("禁用")) -> ()  [unwired: 2 in, 2 out]
          }
        }
        n479 = disable-structure shown="禁用" {
          disable-tunnel: [w999 _] -> w985
          frame Disabled {
            n480 = local read "Microscope"() -> (w1002:enum16{"Miniature", "Benchtop"})
            n481 = Equal?(x=w1002, y=enum16{"Miniature", "Benchtop"}."Benchtop") -> (x = y?=w1000:bool)
            n482 = case shown="真" w1000 {
              tunnel: [FALSE ("Enable") TRUE ("Enable")] -> w999
              frame False {
              }
              frame True {
              }
            }
          }
          frame Enabled {
          }
        }
        n483 = case shown="1" w981 {
          tunnel: w998 -> [w1016 w1056 w1098]
          tunnel: w997 -> [w1015 w1055 w1097]
          tunnel: [w1014 w1048 w1090] -> w996
          tunnel: [w1013 w1047 w1089] -> w991
          tunnel: w994 -> [w1012 w1054 w1096]
          tunnel: w993 -> [w1011 w1053 w1095]
          tunnel: [w1006 w1052 w1094] -> w992
          tunnel: w985 -> [w1005 w1042 w1084]
          tunnel: w977 -> [_ w1041 _]
          frame 0, Default {
            n484 = flat-sequence {
              tunnel: [w1025] -> w1010
              tunnel: [w1024] -> w1009
              tunnel: [w1019] -> w1008
              tunnel: [w1018] -> w1007
              tunnel: w1016 -> [w1021]
              tunnel: w1015 -> [w1020]
              tunnel: w1012 -> [w1025]
              tunnel: w1011 -> [w1024]
              tunnel: [w1040] -> w1014
              tunnel: [w1039] -> w1013
              tunnel: [w1036] -> w1006
              tunnel: w1010 -> [w1038]
              tunnel: w1009 -> [w1037]
              tunnel: w1008 -> [w1035]
              tunnel: w1007 -> [w1034]
              tunnel: w1005 -> [_]
              frame #0 {
                n485 = local write "Focus Flag"(FALSE ("Focus Flag")) -> ()
                n486 = xnode "读取/写入控件"("FPGA VI引用输入"=w1021, "错误输入"=w1020, "FOCUS"=FALSE ("Stop Write")) -> ("FPGA VI引用输出"=w1019:refnum<k20>, "错误输出"=w1018:errorcluster)
                n487 = Wait (ms)(milliseconds to wait=u32 100 ("等待时间（毫秒）")) -> ()  [unwired: 1 out]
              }
              frame #1 {
                n488 = xnode "读取/写入控件"("FPGA VI引用输入"=w1038, "错误输入"=w1037, "Shutter"=FALSE, "Start Control"=FALSE ("Enable")) -> ("错误输出"=w1036:errorcluster)  [unwired: 1 out]
                n489 = xnode "Invoke Method"("FPGA VI引用输入"=w1035, "错误输入"=w1034, "元素数量"=u32 0, "超时(ms)"=0) -> ("FPGA VI引用输出"=w1032:refnum<k20>, "错误输出"=w1031:errorcluster, "剩余元素"=w1030:u32)  [unwired: 1 out]
                "Test Point 3" <- w1030
                n490 = xnode "Invoke Method"("FPGA VI引用输入"=w1032, "错误输入"=w1031, "元素数量"=w1030, "超时(ms)"=0) -> ("FPGA VI引用输出"=w1040:refnum<k20>, "错误输出"=w1039:errorcluster)  [unwired: 2 out]
              }
            }
          }
          frame 1 {
            n491 = flat-sequence {
              tunnel: w1053 -> [w1060]
              tunnel: w1054 -> [w1063]
              tunnel: w1055 -> [w1064]
              tunnel: w1056 -> [w1065]
              tunnel: [w1065] -> w1046
              tunnel: [w1064] -> w1045
              tunnel: [w1062] -> w1044
              tunnel: [w1061] -> w1043
              tunnel: w1042 -> [_]
              tunnel: w1041 -> [w1057]
              tunnel: [w1066] -> w1051
              tunnel: [w1069] -> w1050
              tunnel: [w1068] -> w1049
              tunnel: w1046 -> [w1069]
              tunnel: w1045 -> [w1068]
              tunnel: w1044 -> [_]
              tunnel: w1043 -> [w1066]
              tunnel: w1051 -> [w1083]
              tunnel: w1050 -> [w1078]
              tunnel: w1049 -> [w1077]
              tunnel: [w1083] -> w1052
              tunnel: [w1075] -> w1048
              tunnel: [w1074] -> w1047
              frame #0 {
                n492 = xnode "读取/写入控件"("FPGA VI引用输入"=w1063, "错误输入"=w1060, "Start Control"=TRUE ("Start"), "Shutter"=w1057) -> ("FPGA VI引用输出"=w1062:refnum<k20>, "错误输出"=w1061:errorcluster)
                n493 = Wait (ms)(milliseconds to wait=u32 100 ("等待时间（毫秒）")) -> ()  [unwired: 1 out]
              }
              frame #1 {
                n494 = local write "Focus Flag"(TRUE ("Focus Flag")) -> ()
              }
              frame #2 {
                n495 = xnode "Invoke Method"("FPGA VI引用输入"=w1078, "错误输入"=w1077, "元素数量"=u32 0, "超时(ms)"=0) -> ("FPGA VI引用输出"=w1081:refnum<k20>, "错误输出"=w1080:errorcluster, "剩余元素"=w1079:u32)  [unwired: 1 out]
                n496 = xnode "Invoke Method"("FPGA VI引用输入"=w1081, "错误输入"=w1080, "元素数量"=w1079, "超时(ms)"=0) -> ("FPGA VI引用输出"=w1073:refnum<k20>, "错误输出"=w1072:errorcluster)  [unwired: 2 out]
                n497 = xnode "读取/写入控件"("FPGA VI引用输入"=w1073, "错误输入"=w1072, "FOCUS"=TRUE ("Stop Write")) -> ("FPGA VI引用输出"=w1075:refnum<k20>, "错误输出"=w1074:errorcluster)
              }
            }
          }
          frame 2 {
            n498 = flat-sequence {
              tunnel: w1095 -> [w1102]
              tunnel: w1096 -> [w1105]
              tunnel: w1097 -> [w1106]
              tunnel: w1098 -> [w1107]
              tunnel: [w1107] -> w1088
              tunnel: [w1106] -> w1087
              tunnel: [w1104] -> w1086
              tunnel: [w1103] -> w1085
              tunnel: w1084 -> [_]
              tunnel: [w1108] -> w1093
              tunnel: [w1111] -> w1092
              tunnel: [w1110] -> w1091
              tunnel: w1088 -> [w1111]
              tunnel: w1087 -> [w1110]
              tunnel: w1086 -> [_]
              tunnel: w1085 -> [w1108]
              tunnel: w1093 -> [w1125]
              tunnel: w1092 -> [w1120]
              tunnel: w1091 -> [w1119]
              tunnel: [w1125] -> w1094
              tunnel: [w1117] -> w1090
              tunnel: [w1116] -> w1089
              frame #0 {
                n499 = xnode "读取/写入控件"("FPGA VI引用输入"=w1105, "错误输入"=w1102, "Start Control"=TRUE ("Start"), "Shutter"=TRUE) -> ("FPGA VI引用输出"=w1104:refnum<k20>, "错误输出"=w1103:errorcluster)
                n500 = Wait (ms)(milliseconds to wait=u32 100 ("等待时间（毫秒）")) -> ()  [unwired: 1 out]
              }
              frame #1 {
                n501 = local write "Focus Flag"(TRUE ("Focus Flag")) -> ()
              }
              frame #2 {
                n502 = xnode "Invoke Method"("FPGA VI引用输入"=w1120, "错误输入"=w1119, "元素数量"=u32 0, "超时(ms)"=0) -> ("FPGA VI引用输出"=w1123:refnum<k20>, "错误输出"=w1122:errorcluster, "剩余元素"=w1121:u32)  [unwired: 1 out]
                n503 = xnode "Invoke Method"("FPGA VI引用输入"=w1123, "错误输入"=w1122, "元素数量"=w1121, "超时(ms)"=0) -> ("FPGA VI引用输出"=w1115:refnum<k20>, "错误输出"=w1114:errorcluster)  [unwired: 2 out]
                n504 = xnode "读取/写入控件"("FPGA VI引用输入"=w1115, "错误输入"=w1114, "FOCUS"=TRUE ("Stop Write")) -> ("FPGA VI引用输出"=w1117:refnum<k20>, "错误输出"=w1116:errorcluster)
              }
            }
          }
        }
        n505 = Merge Errors(w992, w991) -> (w990:errorcluster)
      }
      event "Z-Stack": Value Change {
        n506 = event-data() -> ()  [unwired: 1 in, 6 out]
        n507 = disable-structure shown="禁用" {
          disable-tunnel: [w1147 _] -> w1133
          frame Disabled {
            n508 = local read "Microscope"() -> (w1148:enum16{"Miniature", "Benchtop"})
            n509 = Equal?(x=w1148, y=enum16{"Miniature", "Benchtop"}."Benchtop") -> (x = y?=w1150:bool)
            n510 = case shown="假" w1150 {
              tunnel: [FALSE ("Enable") TRUE ("Enable")] -> w1147
              frame False {
              }
              frame True {
              }
            }
          }
          frame Enabled {
          }
        }
        n511 = case shown="真" "Z-Stack" {
          tunnel: w1146 -> [w1171 w1242]
          tunnel: w1145 -> [w1170 w1241]
          tunnel: [w1169 w1234] -> w1144
          tunnel: [w1168 w1233] -> w1139
          tunnel: w1142 -> [w1167 w1240]
          tunnel: w1141 -> [w1166 w1239]
          tunnel: [w1161 w1238] -> w1140
          tunnel: w1136 -> [w1157 w1225]
          tunnel: [w1154 w1228] -> w1135
          tunnel: w1133 -> [_ w1224]
          frame False {
            n512 = flat-sequence {
              tunnel: [w1181] -> w1165
              tunnel: [w1180] -> w1164
              tunnel: [w1175] -> w1163
              tunnel: [w1174] -> w1162
              tunnel: w1171 -> [w1177]
              tunnel: w1170 -> [w1176]
              tunnel: w1167 -> [w1181]
              tunnel: w1166 -> [w1180]
              tunnel: w1157 -> [w1172]
              tunnel: [w1172] -> w1156
              tunnel: w1165 -> [w1195]
              tunnel: w1164 -> [w1194]
              tunnel: w1163 -> [w1192]
              tunnel: w1162 -> [w1191]
              tunnel: [w1197] -> w1160
              tunnel: [w1196] -> w1159
              tunnel: [w1193] -> w1158
              tunnel: w1156 -> [w1183]
              tunnel: [w1183] -> w1155
              tunnel: [w1182] -> w1153
              tunnel: [w1199] -> w1161
              tunnel: [w1203] -> w1168
              tunnel: [w1205] -> w1169
              tunnel: w1160 -> [w1204]
              tunnel: w1159 -> [w1202]
              tunnel: w1158 -> [w1200]
              tunnel: w1155 -> [w1209]
              tunnel: [w1207] -> w1154
              tunnel: w1153 -> [w1201]
              frame #0 {
                n513 = local write "Focus Flag"(FALSE ("Focus Flag")) -> ()
                n514 = xnode "读取/写入控件"("FPGA VI引用输入"=w1177, "错误输入"=w1176, "FOCUS"=FALSE ("Stop Write")) -> ("FPGA VI引用输出"=w1175:refnum<k20>, "错误输出"=w1174:errorcluster)
                n515 = Wait (ms)(milliseconds to wait=u32 50 ("等待时间（毫秒）")) -> ()  [unwired: 1 out]
              }
              frame #1 {
                n516 = xnode "Invoke Method"("FPGA VI引用输入"=w1192, "错误输入"=w1191, "元素数量"=u32 0, "超时(ms)"=0) -> ("FPGA VI引用输出"=w1189:refnum<k20>, "错误输出"=w1188:errorcluster, "剩余元素"=w1187:u32)  [unwired: 1 out]
                n517 = xnode "读取/写入控件"("FPGA VI引用输入"=w1195, "错误输入"=w1194, "Start Control"=FALSE ("Enable")) -> ("FPGA VI引用输出"=w1182:refnum<k20>, "错误输出"=w1193:errorcluster)
                n518 = xnode "Invoke Method"("FPGA VI引用输入"=w1189, "错误输入"=w1188, "元素数量"=w1187, "超时(ms)"=0) -> ("FPGA VI引用输出"=w1197:refnum<k20>, "错误输出"=w1196:errorcluster)  [unwired: 2 out]
              }
              frame #2 {
                n519 = local read "Slices"() -> (w1198:u16)
                n520 = Increment(x=w1209) -> (x+1=w1206:u16)
                n521 = Greater Or Equal?(x=w1206, y=w1198) -> (x >= y?=w1208:bool)
                n522 = case shown="假" w1208 {
                  tunnel: [w1213 u16 0] -> w1207
                  tunnel: w1206 -> [w1213 _]
                  tunnel: [w1212 w1219] -> w1205
                  tunnel: w1204 -> [w1212 w1219]
                  tunnel: [w1211 w1220] -> w1203
                  tunnel: w1202 -> [w1211 w1220]
                  tunnel: w1201 -> [_ w1217]
                  tunnel: w1200 -> [w1210 w1216]
                  tunnel: [w1210 w1215] -> w1199
                  frame False {
                    n523 = property on="Move" class="Bool (严格)"("Val(Sgnl)"=TRUE ("值(信号)")) -> ()  [unwired: 2 in, 2 out]
                  }
                  frame True {
                    n524 = xnode "读取/写入控件"("FPGA VI引用输入"=w1217, "错误输入"=w1216, "Shutter"=FALSE ("Enable")) -> ("错误输出"=w1215:errorcluster)  [unwired: 1 out]
                    n525 = property on="Save" class="Bool (严格)"("DisabledEnum"=T4."Enabled" ("禁用")) -> ()  [unwired: 2 in, 2 out]
                    n526 = property on="LIVE" class="Bool (严格)"("DisabledEnum"=T4."Enabled" ("禁用")) -> ()  [unwired: 2 in, 2 out]
                  }
                }
              }
            }
          }
          frame True {
            n527 = flat-sequence {
              tunnel: w1239 -> [w1246]
              tunnel: w1240 -> [w1249]
              tunnel: w1241 -> [w1250]
              tunnel: w1242 -> [w1251]
              tunnel: [w1251] -> w1232
              tunnel: [w1250] -> w1231
              tunnel: [w1248] -> w1230
              tunnel: [w1247] -> w1229
              tunnel: [w1245] -> w1226
              tunnel: w1225 -> [w1245]
              tunnel: w1224 -> [_]
              tunnel: [w1253] -> w1237
              tunnel: [w1256] -> w1236
              tunnel: [w1255] -> w1235
              tunnel: w1232 -> [w1256]
              tunnel: w1231 -> [w1255]
              tunnel: w1230 -> [_]
              tunnel: w1229 -> [w1253]
              tunnel: [w1252] -> w1227
              tunnel: w1226 -> [w1252]
              tunnel: w1237 -> [w1271]
              tunnel: w1236 -> [w1266]
              tunnel: w1235 -> [w1265]
              tunnel: [w1271] -> w1238
              tunnel: [w1263] -> w1234
              tunnel: [w1262] -> w1233
              tunnel: [w1257] -> w1228
              tunnel: w1227 -> [w1257]
              frame #0 {
                w1243 = TRUE ("Start")
                n528 = xnode "读取/写入控件"("FPGA VI引用输入"=w1249, "错误输入"=w1246, "Start Control"=w1243, "Shutter"=w1243) -> ("FPGA VI引用输出"=w1248:refnum<k20>, "错误输出"=w1247:errorcluster)
                n529 = Wait (ms)(milliseconds to wait="Interval Time") -> ()  [unwired: 1 out]
              }
              frame #1 {
                n530 = local write "Focus Flag"(TRUE ("Focus Flag")) -> ()
              }
              frame #2 {
                n531 = xnode "Invoke Method"("FPGA VI引用输入"=w1266, "错误输入"=w1265, "元素数量"=u32 0, "超时(ms)"=0) -> ("FPGA VI引用输出"=w1269:refnum<k20>, "错误输出"=w1268:errorcluster, "剩余元素"=w1267:u32)  [unwired: 1 out]
                n532 = xnode "Invoke Method"("FPGA VI引用输入"=w1269, "错误输入"=w1268, "元素数量"=w1267, "超时(ms)"=0) -> ("FPGA VI引用输出"=w1261:refnum<k20>, "错误输出"=w1260:errorcluster)  [unwired: 2 out]
                n533 = xnode "读取/写入控件"("FPGA VI引用输入"=w1261, "错误输入"=w1260, "FOCUS"=TRUE ("Stop Write")) -> ("FPGA VI引用输出"=w1263:refnum<k20>, "错误输出"=w1262:errorcluster)
              }
            }
          }
        }
        n534 = case shown="真" "Z-Stack" {
          frame False {
          }
          frame True {
          }
        }
        n535 = Merge Errors(w1140, w1139) -> (w1138:errorcluster)
      }
      event "Pixel/Line", "Line": Value Change {
        n536 = event-data() -> ()  [unwired: 1 in, 6 out]
        n537 = xnode "读取/写入控件"("FPGA VI引用输入"=w1286, "错误输入"=w1285, "FOCUS"=FALSE) -> ("FPGA VI引用输出"=w1279:refnum<k20>, "错误输出"=w1276:errorcluster)
        n538 = flat-sequence {
          tunnel: w1279 -> [w1301]
          tunnel: [w1301] -> w1278
          tunnel: [w1300] -> w1277
          tunnel: w1276 -> [w1300]
          frame #0 {
            n539 = Wait (ms)(milliseconds to wait=u32 5 ("等待时间（毫秒）")) -> ()  [unwired: 1 out]
          }
        }
        n540 = xnode "Invoke Method"("FPGA VI引用输入"=w1278, "错误输入"=w1277, "元素数量"=u32 0, "超时(ms)"=0) -> ("FPGA VI引用输出"=w1289:refnum<k20>, "错误输出"=w1290:errorcluster, "剩余元素"=w1287:u32)  [unwired: 1 out]
        n541 = xnode "Invoke Method"("FPGA VI引用输入"=w1289, "错误输入"=w1290, "元素数量"=w1287, "超时(ms)"=0) -> ("FPGA VI引用输出"=w1275:refnum<k20>, "错误输出"=w1274:errorcluster)  [unwired: 2 out]
        n542 = local read "LIVE"() -> (w1272:bool)
        n543 = case shown="假" w1272 {
          tunnel: [w1294 w1298] -> w1283
          tunnel: [w1293 w1297] -> w1282
          tunnel: w1275 -> [w1294 w1296]
          tunnel: w1274 -> [w1293 w1295]
          frame False {
          }
          frame True {
            n544 = xnode "读取/写入控件"("FPGA VI引用输入"=w1296, "错误输入"=w1295, "FOCUS"=TRUE) -> ("FPGA VI引用输出"=w1298:refnum<k20>, "错误输出"=w1297:errorcluster)
          }
        }
      }
      event "Stop": Value Change {
        n545 = event-data() -> ()  [unwired: 1 in, 3 out]
        n546 = xnode "Invoke Method"("FPGA VI引用输入"=w1313, "错误输入"=w1312) -> ("FPGA VI引用输出"=w1307:refnum<k20>, "错误输出"=w1306:errorcluster)
        n547 = xnode "Invoke Method"("FPGA VI引用输入"=w1307, "错误输入"=w1306) -> ("FPGA VI引用输出"=w1305:refnum<k20>, "错误输出"=w1304:errorcluster)
        n548 = xnode "Invoke Method"("FPGA VI引用输入"=w1305, "错误输入"=w1304) -> ("FPGA VI引用输出"=w1315:refnum<k20>, "错误输出"=w1314:errorcluster)
        "Power Stop" <- TRUE ("Power Stop")
      }
    }
  }
  n549 = local read "Rolling Average"() -> (w33:dbl)
  n550 = Obtain Queue(max queue size (-1, unlimited)=w33, name (unnamed)="Rolling Init" ("名称（未命名）"), element data type=dbl[][] [] ("x/y")) -> (queue out=w45:refnum<queue>, error out=w46:errorcluster)  [unwired: 2 in, 1 out]
  n551 = call "IMAQ Create"("Image Name"="ROI Mask", "Image Type"=w3) -> ("New Image"=w2:T1, "error out"=w1:errorcluster)  [unwired: 3 in]
  n552 = call "IMAQ Create"("Image Name"="Rolling", "Image Type"=w35) -> ("New Image"=w39:T1)  [unwired: 3 in, 1 out]
  n553 = call "IMAQ Create"("Image Name"="Display-IMAQ", "Image Type"=w9) -> ("New Image"=w8:T1)  [unwired: 3 in, 1 out]
  n554 = call "IMAQ Create"("Image Name"="92", "Image Type"=w15) -> ("New Image"=w13:T1, "error out"=w12:errorcluster)  [unwired: 3 in]
  n555 = Initialize Array(0.0 ("元素"), w38, w38) -> (w36:dbl[][])
  n556 = while {
    shift-right: [w1333] -> _
    shift-left: w36 -> [w1334]
    tunnel: w39 -> [w1332]
    shift-right: [w1331] -> w40
    shift-left: w45 -> [w1329]
    shift-right: [w1330] -> w41
    shift-left: w46 -> [w1328]
    shift-right: [w1327] -> _
    shift-left: 1.0 ("Rolling Average") -> [w1326]
    tunnel: w21 -> [w1324]
    shift-right: [w1321] -> _
    shift-left: u16 0 -> [w1322]
    tunnel: w13 -> [w1320]
    tunnel: w12 -> [w1319]
    tunnel: w8 -> [w1318]
    tunnel: w2 -> [w1317]
    tunnel: w1 -> [w1316]
    i -> [w1325]
    stop <- w1337 stop-if-true
    n557 = Dequeue Element(queue=w1324) -> (queue out=w1323:refnum<queue>, element=w1335:i16[][], error out=w1336:errorcluster)  [unwired: 2 in, 1 out]
    n558 = case shown="无错误" w1336 {
      tunnel: [_ TRUE] -> w1337
      tunnel: w1335 -> [w1340 _]
      tunnel: w1334 -> [w1358 _]
      tunnel: [w1345 dbl[][] [] ("x/y")] -> w1333
      tunnel: w1332 -> [w1353 _]
      tunnel: [w1363 w1432] -> w1331
      tunnel: [w1356 w1431] -> w1330
      tunnel: w1329 -> [w1361 w1432]
      tunnel: w1328 -> [w1360 w1431]
      tunnel: [w1359 w1430] -> w1327
      tunnel: w1326 -> [w1362 w1430]
      tunnel: w1325 -> [w1357 _]
      tunnel: w1323 -> [w1355 _]
      tunnel: w1322 -> [w1351 _]
      tunnel: [w1350 u16 0] -> w1321
      tunnel: w1320 -> [w1348 _]
      tunnel: w1319 -> [w1347 _]
      tunnel: w1318 -> [w1346 _]
      tunnel: w1317 -> [w1343 _]
      tunnel: w1316 -> [w1341 _]
      frame No Error {
        n559 = Get Queue Status(queue=w1355) -> (# elements in queue=→"Memory":i32)  [unwired: 2 in, 7 out]
        n560 = local read "Pulse Number"() -> (w1338:enum16{"SP", "DP"})
        n561 = Increment(x=w1351) -> (x+1=w1350:u16)
        "Total Frames" <- w1350
        n562 = call "sub_数组奇数行转置.vi"("Pulse Number"=w1338, "Input"=w1340) -> ("output"=w1339:u16[][])
        n563 = case shown="假" "Rolling" {
          tunnel: [w1390 w1410] -> w1345
          tunnel: [w1389 w1409] -> w1363
          tunnel: w1362 -> [w1388 _]
          tunnel: w1361 -> [w1389 w1408]
          tunnel: w1360 -> [w1392 w1407]
          tunnel: [w1388 w1406] -> w1359
          tunnel: w1358 -> [w1390 w1405]
          tunnel: w1357 -> [_ w1404]
          tunnel: [w1391 w1403] -> w1356
          tunnel: w1353 -> [_ w1402]
          tunnel: [w1393 w1400] -> w1344
          tunnel: w1346 -> [w1387 _]
          tunnel: w1339 -> [w1386 w1394]
          frame False {
            n564 = call "IMAQ ArrayToImage"("Image Pixels (U16)"=w1386, "error in (no error)"=w1392, "Image"=w1387) -> ("error out"=w1391:errorcluster, "Image Out"=w1393:T1)  [unwired: 7 in]
          }
          frame True {
            n565 = case shown="真" "Rolling Queue Flag" {
              tunnel: [w1414 w1420] -> w1396
              tunnel: [w1412 w1419] -> w1398
              tunnel: [w1413 w1427] -> w1406
              tunnel: "Rolling Average" -> [w1413 w1427]
              tunnel: w1408 -> [w1414 w1422]
              tunnel: w1407 -> [w1412 w1421]
              tunnel: [w1411 w1424] -> w1397
              tunnel: w1405 -> [w1411 _]
              tunnel: w1404 -> [_ w1416]
              frame False {
              }
              frame True {
                w1425 = 2048 ("维数大小")
                n566 = Release Queue(queue=w1422, error in (no error)=w1421) -> ()  [unwired: 1 in, 3 out]
                n567 = local write "Rolling Queue Flag"(FALSE ("Rolling Queue Flag")) -> ()
                n568 = Number To Decimal String(number=w1416) -> (decimal integer string=w1417:string)  [unwired: 1 in]
                n569 = Obtain Queue(max queue size (-1, unlimited)=w1427, name (unnamed)=w1417, element data type=dbl[][] [] ("x/y")) -> (queue out=w1423:refnum<queue>, error out=w1418:errorcluster)  [unwired: 2 in, 1 out]
                n570 = Initialize Array(0.0 ("元素"), w1425, w1425) -> (w1424:dbl[][])
                n571 = Flush Queue(queue=w1423, error in (no error)=w1418) -> (queue out=w1420:refnum<queue>, error out=w1419:errorcluster)  [unwired: 1 out]
              }
            }
            n572 = call "sub_rolling average.vi"("Raw Data"=w1394, "错误输入（无错误）"=w1398, "队列输入"=w1396, "移位in"=w1397, "Image Create"=w1402) -> ("错误输出"=w1403:errorcluster, "队列输出"=w1409:refnum<queue>, "移位out"=w1410:dbl[][], "Image Display"=w1400:T1, "队列中元素数量"=→"Queue Number":i32)  [unwired: 2 in]
          }
        }
        "Image" <- w1344
        n573 = case shown="真" "Read offset" {
          tunnel: w1344 -> [_ w1381]
          tunnel: w1343 -> [_ w1382]
          tunnel: w1341 -> [_ w1380]
          frame False {
          }
          frame True {
            n574 = property on="Image" class="ImageControl"() -> ("ROI"=w1383:T5)  [unwired: 2 in, 2 out]
            n575 = call "ROI统计量16bit.vi"("error in (no error)"=w1380, "ROI Descriptor"=w1383, "Image Mask"=w1382, "Image"=w1381) -> ("统计量"=w1384:sgl[])  [unwired: 5 in, 2 out]
            n576 = Index Array(array=w1384, index=0 ("索引")) -> (element=w1379:sgl)
            "波形图表" <- w1379
            n577 = To Word Integer(number=w1379) -> (16bit integer=→"Offset value":i16)
          }
        }
        n578 = case shown="真" "Calculate Phase shift" {
          tunnel: w1344 -> [_ w1368]
          tunnel: w1348 -> [_ w1367]
          tunnel: w1347 -> [_ w1366]
          frame False {
          }
          frame True {
            n579 = property on="Image" class="ImageControl"() -> ("ROI"=w1371:T5)  [unwired: 2 in, 2 out]
            n580 = Unbundle By Name(w1371) -> ("Global Rectangle"=w1373:i32[])
            n581 = call "sub_转换成偶数数组.vi"("输入数组"=w1373) -> ("输出数组"=w1372:i32[])
            n582 = call "IMAQ Extract 2"("Optional Rectangle"=w1372, "error in (no error)"=w1366, "Image Dst"=w1367, "Image Src"=w1368) -> ("error out"=w1375:errorcluster, "Image Dst Out"=w1374:T1)  [unwired: 6 in]
            n583 = call "IMAQ ImageToArray"("error in (no error)"=w1375, "Image"=w1374) -> ("Image Pixels (I16)"=w1364:i16[][])  [unwired: 2 in, 4 out]
            n584 = To Double Precision Float(number=w1364) -> (double precision float=w1365:dbl[][])
            n585 = call "sub_提取奇偶行2.vi"("数组"=w1365) -> ("奇数行一维数组"=w1377:dbl[], "偶数行一维数组"=w1376:dbl[])  [unwired: 5 in]
            n586 = call "sub_互相关.vi"("互相关点数"="互相关点数", "y"=w1376, "x"=w1377) -> ("中心偏移"=→"中心偏移":i32)  [unwired: 2 in, 2 out]
          }
        }
      }
      frame Error {
      }
    }
  }
  n587 = xnode "关闭FPGA VI引用"("FPGA VI引用输入"=w57, "错误输入"=w56) -> ()  [unwired: 1 out]
  n588 = Release Queue(queue=w32, error in (no error)=w73) -> ()  [unwired: 1 in, 3 out]
  n589 = Release Queue(queue=w21, error in (no error)=w20) -> ()  [unwired: 1 in, 3 out]
  n590 = Release Queue(queue=w40, error in (no error)=w41) -> ()  [unwired: 1 in, 3 out]
  n591 = xnode "关闭FPGA VI引用"("FPGA VI引用输入"=w72, "错误输入"=w71) -> ()  [unwired: 1 out]
